vi "DialogCreateClass.vi"(0 "ClassWriterNative.lvclass":refnum<class "ClassWriterNative.lvclass">, 1 "ProjectItem Refnum":refnum<vi>, 5 "error in (no error)":errorcluster) -> (13 "InterfaceToImplement":T3, 14 "Reference out":refnum<class "ClassWriterNative.lvclass">, 15 "Cancelled":bool, 16 "CreateClassData":T4, 17 "DesignPatternsToAddAfterCreation":string[](array[string]), 18 "ChangeProviderRequested":string, 19 "error out":errorcluster)   [LabVIEW 2020, in "ClassWriterNative.lvclass"]
uses:
  <resource>/Framework/Providers/Open_GDS/ClassProviders/Provider_LvNativeClass/ClassWriterNative_class/ClassWriterNative.lvclass
  <resource>/Framework/Providers/Open_GDS/ClassProviders/Provider_BaseClassInterface/CreateClassData.ctl
  <resource>/Framework/Providers/Open_GDS/ClassProviders/Provider_BaseClassInterface/ClassWriter_class/InterfacesToImplement.ctl
  <resource>/Framework/Providers/Open_GDS/ClassProviders/Common/ScriptingFunctions/Scripting_ConnectorPanePatternType.ctl
  <resource>/Framework/Providers/Open_GDS/ClassProviders/Provider_BaseClassInterface/ClassTemplateType.ctl
  <resource>/Framework/Providers/Open_GDS/ClassProviders/Common/InterfaceLibrary/InterfaceInfo.ctl
  <resource>/Framework/Providers/Open_GDS/ClassProviders/Common/LvClass_class/GDSLvClass_ClassMethodInfo.ctl
  <vilib>/Utility/miscctls.llb/LVRectTypeDef.ctl
  <resource>/Framework/Providers/Open_GDS/ClassProviders/Provider_EndevoGOOP400/EndevoG4ProviderName.ctl
  <vilib>/Utility/miscctls.llb/LVPointTypeDef.ctl
  <vilib>/picture/picture.llb/imagedata.ctl
  <vilib>/Utility/miscctls.llb/LVNodeAndColumnTypeDef.ctl
  <vilib>/Utility/miscctls.llb/LVRowAndColumnUnsignedTypeDef.ctl
  dffca1d0-6338-4fa8-b857-2ce53b536d3f.vi
  <resource>/Framework/Providers/Open_GDS/ClassProviders/Provider_BaseClassInterface/ClassWriter_class/ClassWriter.lvclass
  <resource>/Framework/Providers/Open_GDS/ClassProviders/Common/InterfaceLibrary/InterfaceLibrary.lvlib
panel:
  in  "Help":bool
  in  "_HelpCreateClass":bool
  out "IconSelection":picture
  out "Icon":picture
  in  "ConnectorPanePattern":T1 caption="Connector Pane" items=["4x4x4", "5x6x5", "6x8x6"]
  in  "ModifyTemplates":bool
  in  "AddDesignPattern":bool caption="DESIGN PATTERN"
  out "ProductPicture":picture
  out "TriggerSuffixChange":string
  in  "_CurrentClassProvider":u16(ring) caption="Class Provider To Use" items=["EndevoGOOP300", "Endevo LabVIEW Native", "EndevoGOOP400", "OpenG100"]
  in  "_UseLLB":bool
  out "DupPath":bool
  in  "_ClassType":i32(listbox) caption="Class Templates"
  in  "_ClassFolderSuffix":string caption="Class Folder Suffix"
  in  "_ClassName":string caption="Class Name"
  in  "_ClassDescription":string caption="Class Description"
  in  "_ClassFolder":path caption="Save Class To.."
  in  "_SelectParentClass":string(tree)="Derived Class" caption="Select Parent Class"
  in  "CreateInterfaceMethods":T2(ring)
  in  "InterfaceFilter":string caption="Filter"
  in  "_SelectInterfaceClass":i32[](listbox) caption="Select Parent Interface(s) (ctrl+click to do multiple Selection)"
  in  "_Cancel":bool
  in  "_CreateClass":bool
  out "DesignPatternDescription":string caption="Design Pattern Description"
  in  "DesignPatternList":i32(listbox) caption="Design Patterns"
  # "DESIGN PATTERNS SELECTION"
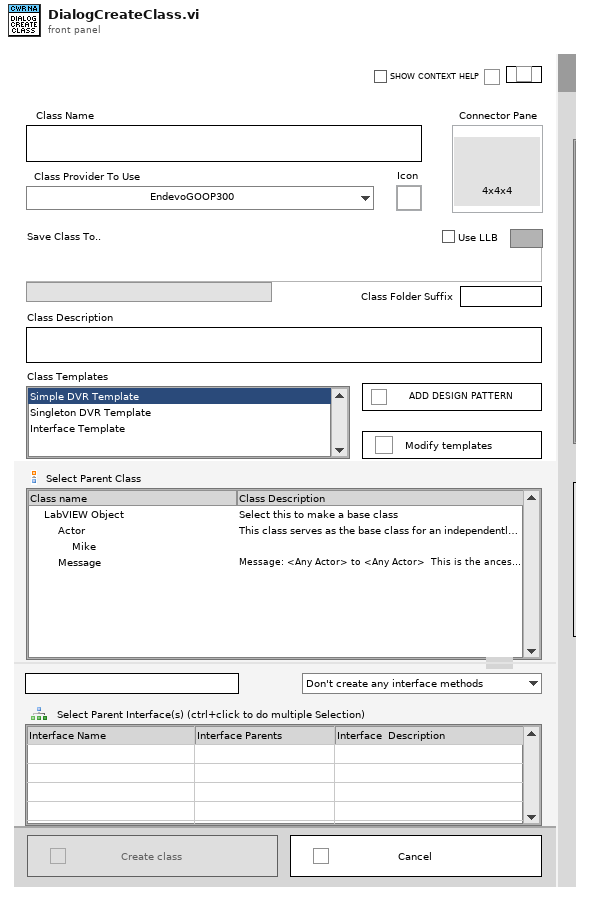
[diagram p1: front panel]
types:
  T1 = typedef "Scripting_ConnectorPanePatternType.ctl" = u16
  T2 = enum16{"Don't create any interface methods", "Create some interface methods", "Create all interface methods"}
  T3 = typedef "ClassWriter.lvclass/InterfacesToImplement.ctl" = cluster{"InterfacePath":path[], "CreateMethods":bool, "MethodsPerInterface(Empty=>All)":cluster{"Methods":string[]}[]}
  T4 = typedef "ClassWriter.lvclass/CreateClassData.ctl" = cluster{"ClassName":string, "ClassFolder":path, "ClassDescription":string, "ClassTemplateOptions":string, "BaseClass(ProjectStringPath or LvClassFilePath)":variant, "ExtraCreateParameters":variant, "FolderSuffix":string}
  T5 = cluster{"Font Name":string, "Size":u16, "Bold":bool, "Italic":bool, "Underline":bool, "Strikeout":bool, "Color":u32}
  T6 = typedef "LVRectTypeDef.ctl" = cluster{"Left":i16, "Top":i16, "Right":i16, "Bottom":i16}
  T7 = typedef "ClassWriter.lvclass/ClassTemplateType.ctl" = cluster{"TemplateIdName":string, "TemplateUserDialogName":string, "OnlySubClassTemplate":bool, "CanDeriveFromTheseTemplateIDs":string[], "ClassSuffix":string, "Description":string, "LvLibTemplate":bool}
  T8 = typedef "InterfaceLibrary.lvlib/InterfaceInfo.ctl" = cluster{"Name(Short if no Conflicts)":string, "FullQualifierName":string, "Description":string, "Path":path, "ParentInterfaceNames(Short if no Conflitcs)":string[], "ParentInterfaceFullQualifierNames":string[], "IconPath":path, "Methods":T9[]}
  T9 = typedef "GDSLvClass_ClassMethodInfo.ctl" = cluster{"Name":string, "Descriptions":string, "RelativePath":path, "SourceScope":enum32{"invalid scope", "public", "private", "protected", "community"}, "MustOverride":bool, "VirtualFolderLocation":string[]}
  T10 = cluster{"Cancel":bool, "OtherTemplates":string[], "BaseClasses":path[], "Templates":T7[], "BaseObjectTag":string, "ClassType(Template)":string, "BaseClassToUse":path, "DeriveFromClass":path, "OpenG":bool, "Derived":bool, "DeriveFromClassRef":refnum<vi>, "ClassPaths":path[], "DesignPatternsVisible":bool, "ClassProviderName":string, "ClassTemplateUsed":string, "PlugInIDs":string[], "DPDescriptions":string[], "DpDependencies":cluster{"DependenciesID":string[]}[], "DPs":string[], "InitDerived":bool, "ClassFolderSuffix":string, "ChangeProviderTo":string, "ClassTags":string[], "LLB_Allowed":bool, "StartFolder":path, "SplitterMouseDown":bool, "InterfaceIcons":path[], "InterfaceInfo":T8[], "OldBnds":T6, "BondsChanged":bool, "ClassTemplateIndex":i32[], "StartBnds":T6}
  T11 = typedef "EndevoG4ProviderName.ctl" = enum16{"EndevoGOOP400"}
  T12 = typedef "LVPointTypeDef.ctl" = cluster{"Horizontal":i16, "Vertical":i16}
  T13 = typedef "imagedata.ctl" = cluster{"image type":i32, "image depth":i32, "image":u8[], "mask":u8[], "colors":u32[], "Rectangle":cluster{"left":i16, "top":i16, "right":i16, "bottom":i16}}
  T14 = typedef "LVNodeAndColumnTypeDef.ctl" = cluster{"Node":string, "Column":i32}
  T15 = typedef "LVRowAndColumnUnsignedTypeDef.ctl" = cluster{"Row":u32, "Column":u32}
  T16 = enum8{"Enabled", "Disabled", "Disabled and Grayed Out"}
  T17 = typedef "GDSLvCLass_ClassSettingsType.ctl" = cluster{"ClassProviderName":string, "ClassTemplateUsed":string, "ClassTemplateVersion":string, "ClassDescription":string, "PlugIns":T18[], "ConnectorPanePattern":string}
  T18 = typedef "GDSLvClass_PlugIn.ctl" = cluster{"Type":T19, "ID":string, "Version":string, "Path":path, "Name":string, "Data":variant}
  T19 = typedef "GDSLvClass_PlugInTypes.ctl" = enum16{"DesignPattern", "MethodTypes"}
  T20 = typedef "BaseProvider_IniFileSettings.ctl" = cluster{"ClassFolderSuffix":string, "InterfaceFolderSuffix":string, "InterfaceIcon":string}
  T21 = enum32{"Invalid", "Standard", "Closed", "Hidden", "Minimized", "Maximized"}
  T22 = typedef "GOOP_WireConfigurationType.ctl" = cluster{"Edge thickness":i32, "Edge color":u32, "Center thickness":i32, "Center pattern":T23, "CenterColor1":u32, "CenterColor2":u32, "Tunnels and terminals colors":u32}
  T23 = typedef "GOOP_WirePattern.ctl" = enum16{"Solid", "Large dash", "Small dash"}
  T24 = typedef "LVPoint32TypeDef.ctl" = cluster{"Horizontal":i32, "Vertical":i32}
  T25 = typedef "DesignPatternsData.ctl" = cluster{"Type":string, "Patterns":cluster{"ID":string, "Path":path, "Name":string, "Desc":string, "Version":string, "DependenciesID":string[], "OnlyOne":bool}[]}
  T26 = cluster{"ID":string, "Path":path, "Name":string, "Desc":string, "Version":string, "DependenciesID":string[], "OnlyOne":bool}[]
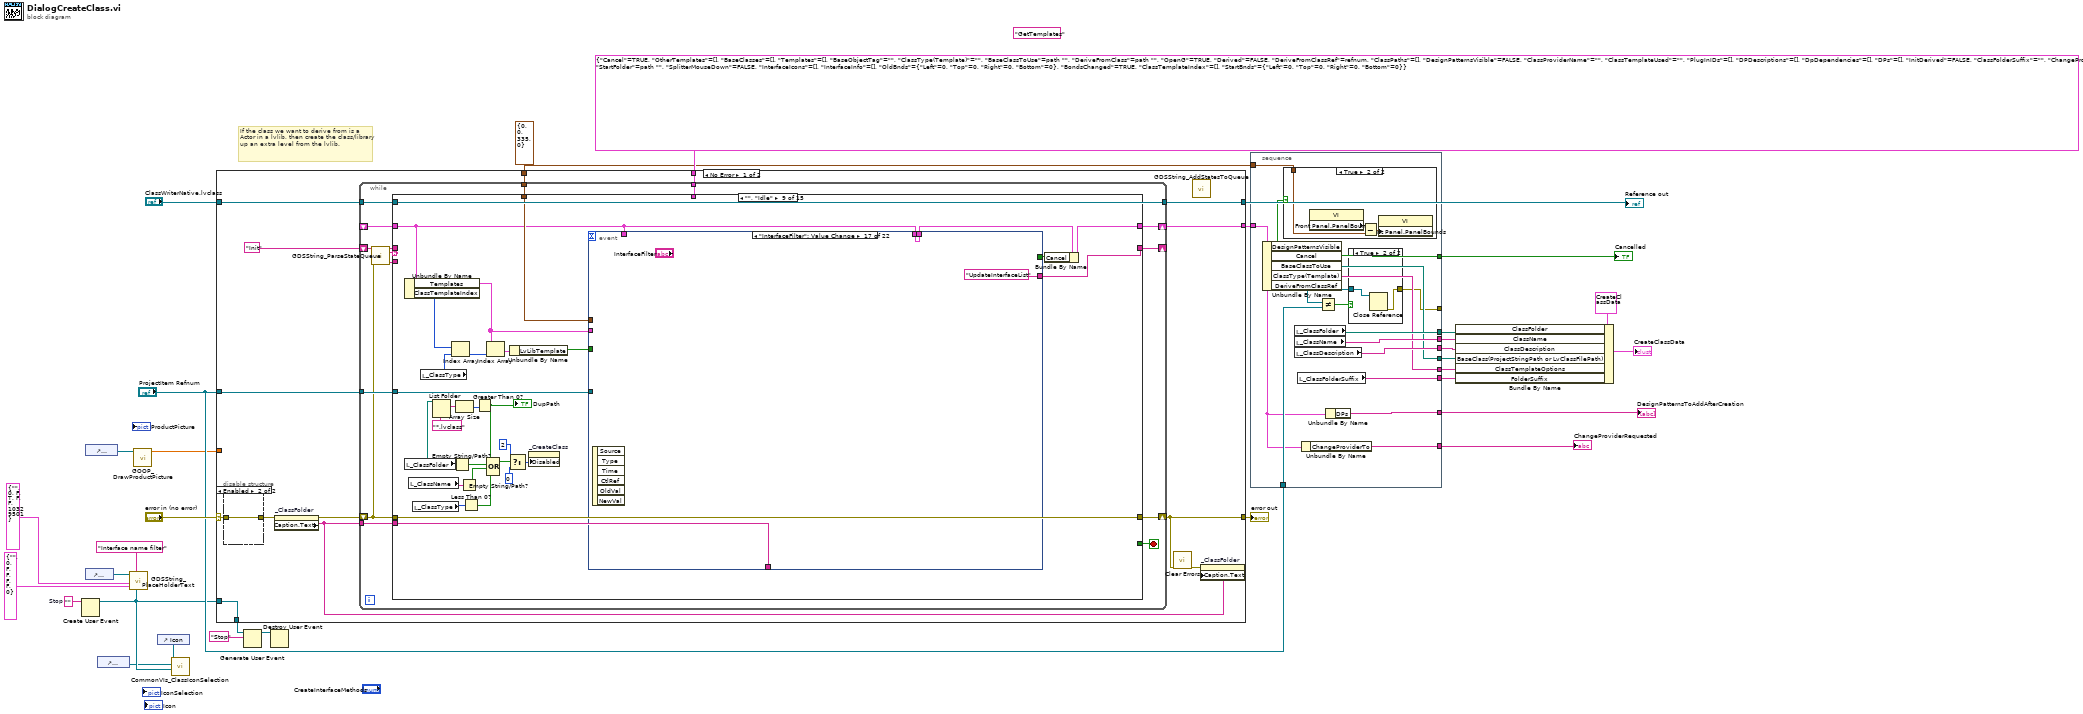
[diagram p0: block diagram]
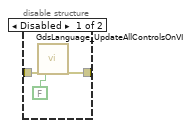
[diagram p4: hidden frame]
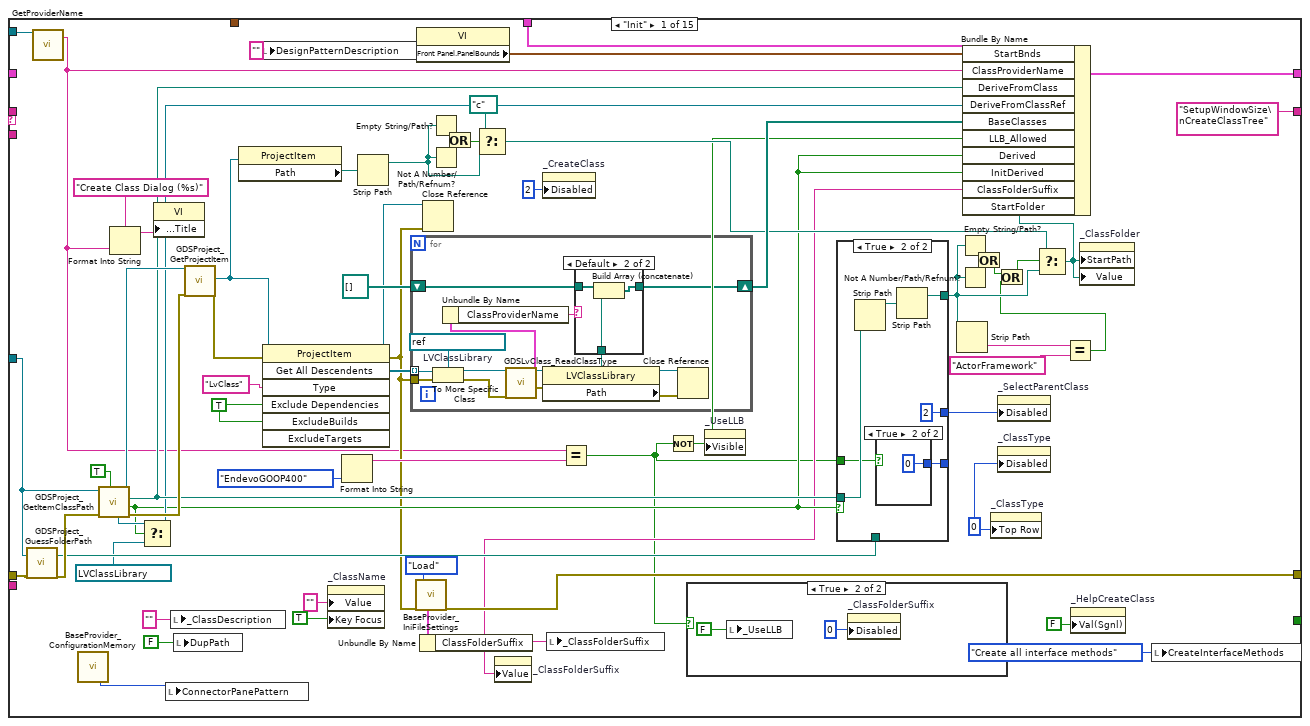
[diagram p5: hidden frame]
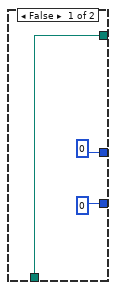
[diagram p8: hidden frame]
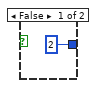
[diagram p9: hidden frame]
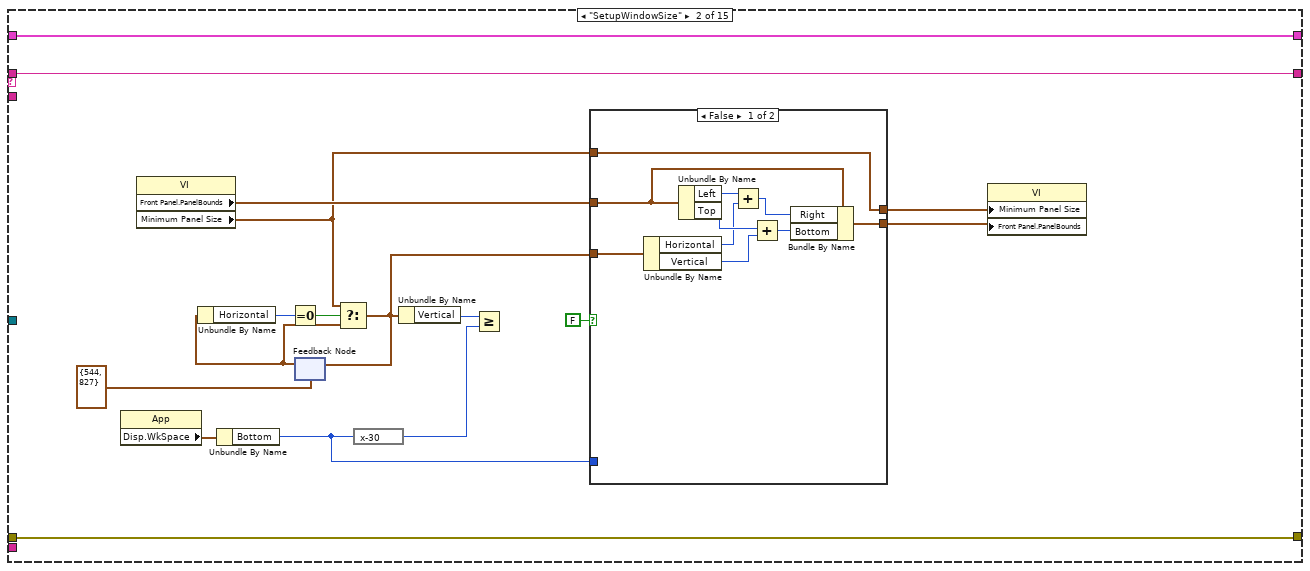
[diagram p10: hidden frame]
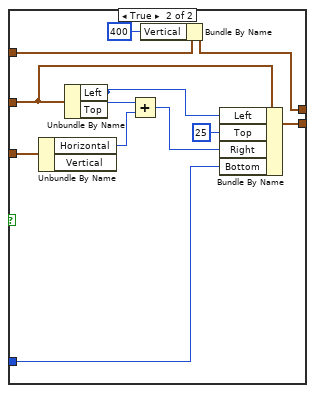
[diagram p11: hidden frame]
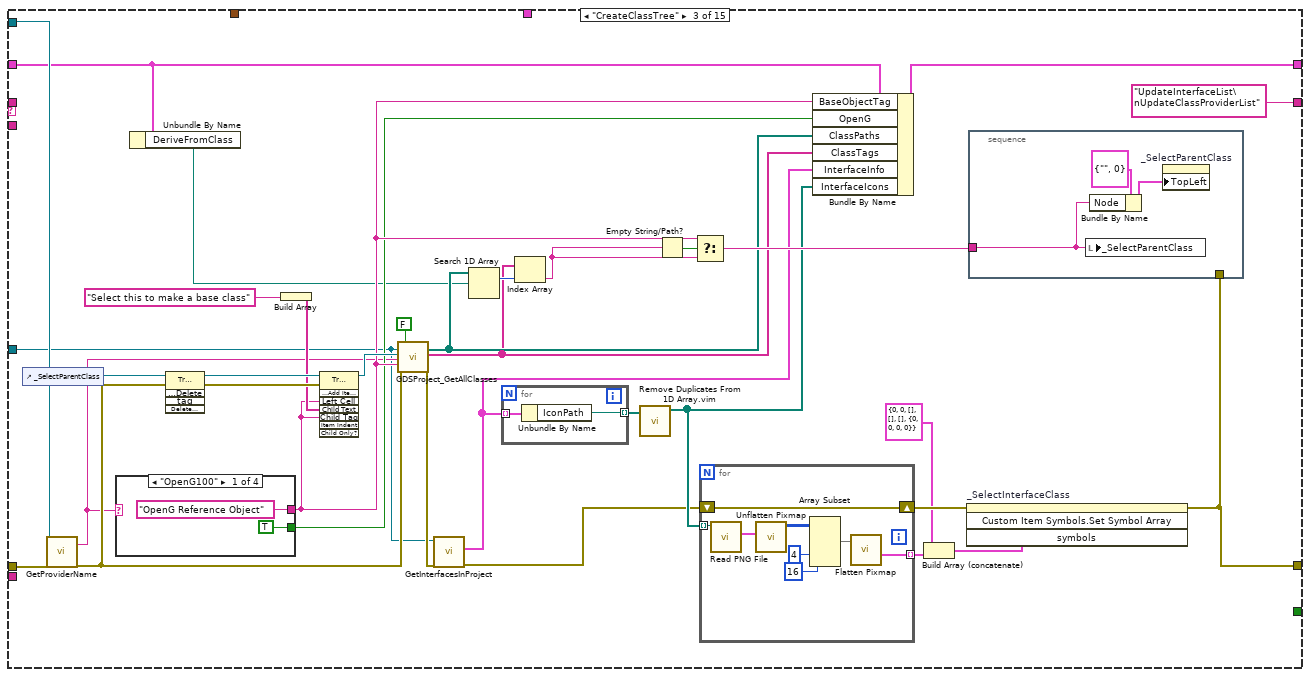
[diagram p12: hidden frame]
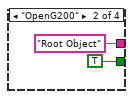
[diagram p13: hidden frame]
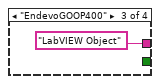
[diagram p14: hidden frame]
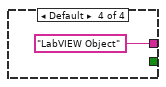
[diagram p15: hidden frame]
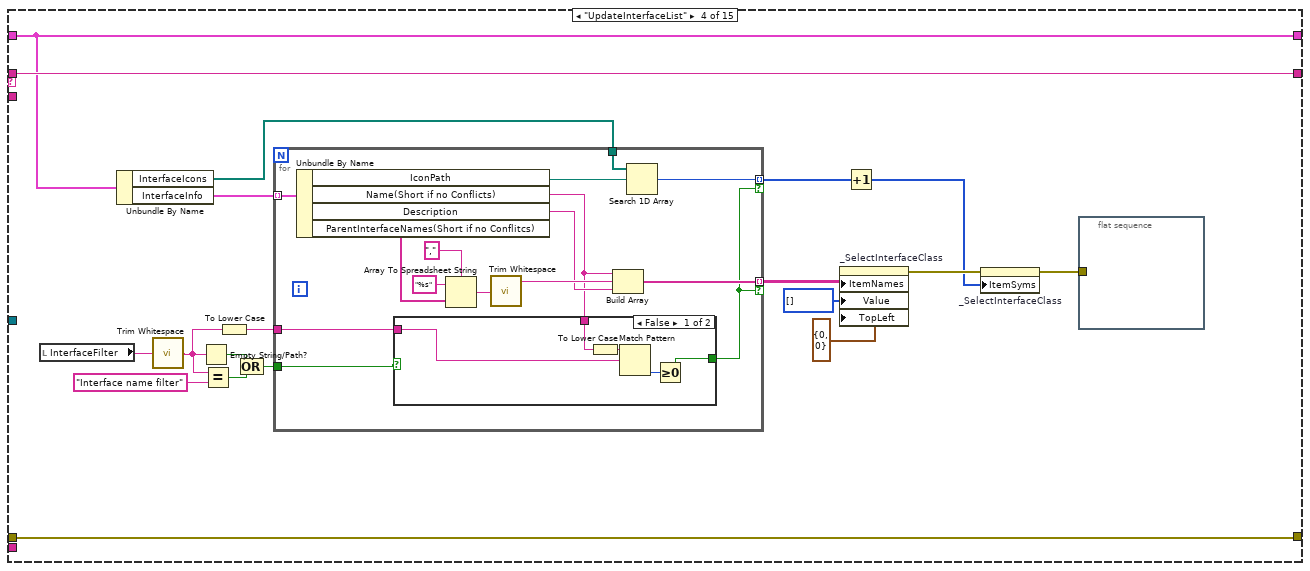
[diagram p16: hidden frame]
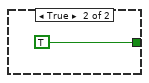
[diagram p17: hidden frame]
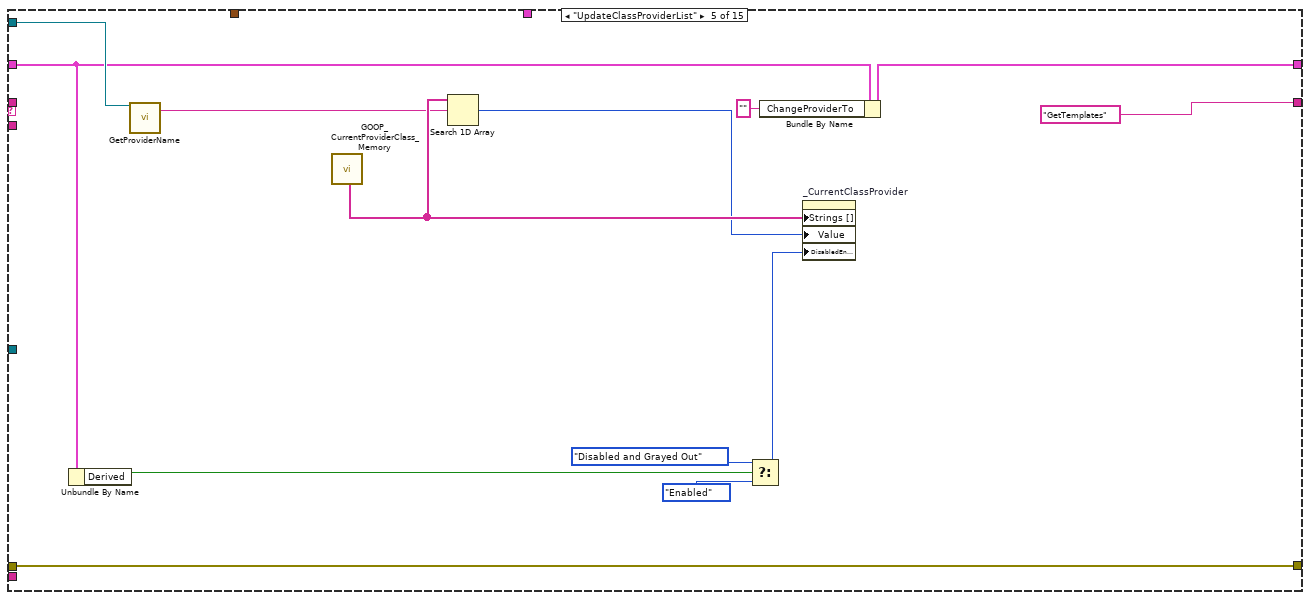
[diagram p18: hidden frame]
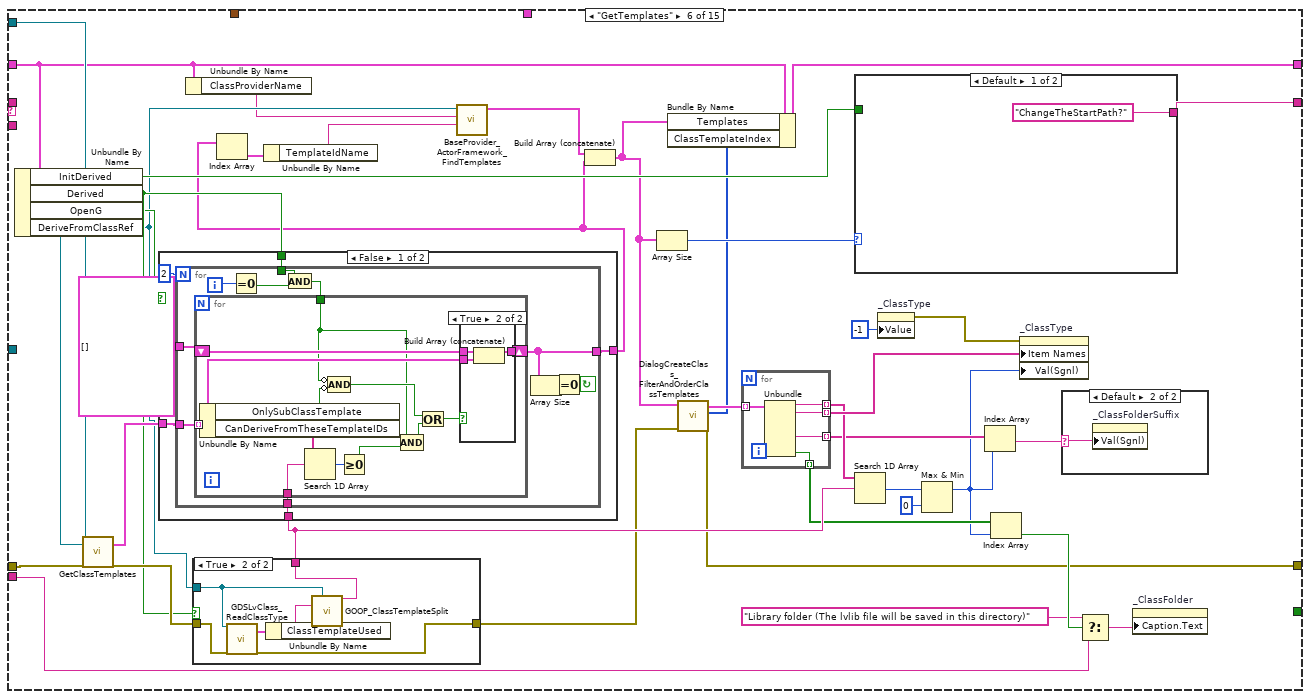
[diagram p19: hidden frame]
diagram:
  w2 = ""  # Stop
  w17 = T6 {"Left"=0, "Top"=0, "Right"=335, "Bottom"=0} ("Rect")
  (unwired) "GetTemplates"
  # "If the class we want to derive from is a\nActor in a lvlib, then create the class/library\nup an extra level from the lvlib."
  n1 = Create User Event(user event datatype=w2) -> (user event=w5:refnum<user-event>)  [unwired: 1 in, 1 out]
  n2 = control-ref of="InterfaceFilter"() -> (w11:refnum<vi>)
  n3 = control-ref of="ProductPicture"() -> (w13:refnum<vi>)
  n4 = control-ref of="IconSelection"() -> (w3:refnum<vi>)
  n5 = call <resource>:"GDSString_PlaceHolderText.vi"("BooleanUserEventToStopPlaceHolderVI"=w5, "PlaceholderText"="Interface name filter" ("InterfaceFilter"), "PlaceholderTextFont(Grey,Italic)"=T5 {"Font Name"="", "Size"=0, "Bold"=FALSE, "Italic"=TRUE, "Underline"=FALSE, "Strikeout"=FALSE, "Color"=10329501}, "NormalTextFont(Black)"=T5 {"Font Name"="", "Size"=0, "Bold"=FALSE, "Italic"=FALSE, "Underline"=FALSE, "Strikeout"=FALSE, "Color"=0}, "PlaceholderStringRef"=w11) -> ()  [unwired: 6 in, 1 out]
  n6 = call <resource>:"GOOP_DrawProductPicture.vi"("ProductPictureControl"=w13) -> ("Zoom Factor"=w12:sgl)  [unwired: 10 in]
  n7 = control-ref of="Icon"() -> (w4:refnum<vi>)
  n8 = call <resource>:"CommonVIs_ClassIconSelection.vi"("Icon"=w4, "Messages(Stop or Empty string will stop this VI)"=w5, "IconSelection"=w3) -> ()  [unwired: 9 in]
  n9 = case shown="No Error" "error in (no error)" {
    selector: "error in (no error)" -> [w41 w1013]
    tunnel: "ClassWriterNative.lvclass" -> [w45 w1012]
    tunnel: [w34 w1013] -> w31
    tunnel: [w46 w1012] -> w29
    tunnel: T10 {"Cancel"=TRUE, "OtherTemplates"=[], "BaseClasses"=[], "Templates"=[], "BaseObjectTag"="", "ClassType(Template)"="", "BaseClassToUse"=path "", "DeriveFromClass"=path "", "OpenG"=TRUE, "Derived"=FALSE, "DeriveFromClassRef"=refnum, "ClassPaths"=[], "DesignPatternsVisible"=FALSE, "ClassProviderName"="", "ClassTemplateUsed"="", "PlugInIDs"=[], "DPDescriptions"=[], "DpDependencies"=[], "DPs"=[], "InitDerived"=FALSE, "ClassFolderSuffix"="", "ChangeProviderTo"="", "ClassTags"=[], "LLB_Allowed"=FALSE, "StartFolder"=path "", "SplitterMouseDown"=FALSE, "InterfaceIcons"=[], "InterfaceInfo"=[], "OldBnds"={"Left"=0, "Top"=0, "Right"=0, "Bottom"=0}, "BondsChanged"=TRUE, "ClassTemplateIndex"=[], "StartBnds"={"Left"=0, "Top"=0, "Right"=0, "Bottom"=0}} ("output cluster") -> [w44 _]
    tunnel: "ProjectItem Refnum" -> [w43 _]
    tunnel: [w42 _] -> w27
    tunnel: w17 -> [w40 _]
    tunnel: w12 -> [_ _]
    tunnel: w5 -> [w36 w1011]
    tunnel: [w36 w1011] -> w8
    frame No Error {
      n10 = disable-structure shown="Enabled" {
        disable-tunnel: w41 -> [w49 w50]
        disable-tunnel: [w47 w50] -> w39
        frame Disabled {
          n11 = call <resource>:"GdsLanguage_UpdateAllControlsOnVI.vi"("error in (no error)"=w49, "CreateLanguageFile(Use this to create a languageFile)"=FALSE) -> ("error out"=w47:errorcluster)  [unwired: 16 in, 1 out]
        }
        frame Enabled {
        }
      }
      n12 = property on="_ClassFolder" class="Path"(error in=w39) -> (error out=w38:errorcluster, "Caption.Text"=w37:string)  [unwired: 1 in, 1 out]
      n13 = while {
        shift-right: [w64] -> w34
        shift-left: w38 -> [w56]
        shift-right: [w54] -> _
        shift-left: "Init" -> [w57]
        shift-right: [w60] -> w42
        shift-left: _ -> [w65]
        tunnel: w45 -> [w63]
        tunnel: [w63] -> w46
        tunnel: w44 -> [w62]
        tunnel: w43 -> [w61]
        tunnel: w40 -> [w59]
        tunnel: w37 -> [w58]
        stop <- w55 stop-if-true
        n14 = call <resource>:"GDSString_ParseStateQueue.vi"("State Queue"=w57, "Error In (no error)"=w56) -> ("Remaining States"=w52:string, "Current State"=w53:string, "Arguments"=w51:string)  [unwired: 9 in, 2 out]
        n15 = case shown="\"\", \"Idle\"" w53 {
          tunnel: w65 -> [_ w176 w221 w267 w293 w320 w401 w427 w434 w809 w838 w899 w984 w1006 w1010]
          tunnel: [w127 w176 w223 w267 w292 w339 w401 w427 w454 w824 w837 w926 w984 w1006 w1010] -> w60
          tunnel: w56 -> [w104 w175 w226 w268 w302 w334 w397 w426 w457 w826 w847 w917 w990 _ w1009]
          tunnel: [w83 w175 w200 w268 w302 w305 w397 w426 w457 w826 w846 w916 w990 errorcluster {"status"=TRUE, "code"=1, "source"="Invalid Case"} ("error out") w1009] -> w64
          tunnel: w63 -> [w96 _ w229 _ w295 w338 _ _ _ _ _ _ _ _ _]
          tunnel: ["SetupWindowSize\nCreateClassTree" w174 "UpdateInterfaceList\nUpdateClassProviderList" w269 "GetTemplates" w340 "Idle" "Idle" w455 w825 "Idle" "GetInterfaceSettings" "Exit" "Exit" "Exit"] -> w54
          tunnel: w62 -> [w126 _ _ _ _ _ _ _ _ _ _ _ _ _ _]
          tunnel: w61 -> [w102 _ w207 _ _ _ _ _ w439 _ _ _ _ _ _]
          tunnel: w59 -> [_ _ _ _ _ _ _ _ w437 _ _ _ _ _ _]
          tunnel: w58 -> [_ _ _ _ _ w313 _ _ w436 w811 _ _ _ _ _]
          tunnel: [_ _ _ _ _ _ _ _ _ _ _ _ _ TRUE TRUE] -> w55
          tunnel: w52 -> [_ w174 _ w269 _ _ _ _ _ w825 _ _ _ _ _]
          tunnel: w51 -> [_ _ _ _ _ _ _ _ _ _ _ _ _ _ _]
          frame "Init" {
            w91 = 0 ("Top Row")
            w95 = TRUE ("ExcludeDependencies")
            n16 = call <resource>:"GDSProject_GuessFolderPath.vi"("ProjectItem"=w102, "error in (no error)"=w104) -> ("Path"=w101:path, "error out"=w103:errorcluster)  [unwired: 14 in, 2 out]
            n17 = call-dynamic "GetProviderName.vi"("ClassWriterNative in"=w96) -> ("ProviderName"=w80:string)  [unwired: 16 in, 2 out]
            n18 = call <resource>:"BaseProvider_ConfigurationMemory.vi"() -> ("PatternOut"=w67:T1)  [unwired: 13 in, 6 out]
            n19 = call <resource>:"GDSProject_GetItemClassPath.vi"("ReturnRefToClass(False)"=TRUE, "error in"=w103, "ProjectItemRefIn"=w102) -> ("error out"=w123:errorcluster, "LvCLassFound"=w86:bool, "Path"=w99:path, "ProjectItemRefOut"=w121:refnum<vi>, "LvClassRef"=w90:refnum<vi>)  [unwired: 3 in, 1 out]
            n20 = Format Into String(format string="Create Class Dialog (%s)", w80) -> (resulting string=w98:string)  [unwired: 2 in, 1 out]
            n21 = Select(t=w90, s=w86, f=refnum<vi> refnum) -> (s? t:f=w89:refnum<vi>)
            n22 = property class="VI"("Front Panel.Title"=w98) -> ()  [unwired: 2 in, 2 out]
            n23 = local write "ConnectorPanePattern"(w67) -> ()
            n24 = local write "_ClassDescription"("" ("Class description")) -> ()
            n25 = local write "DupPath"(FALSE ("DupPath")) -> ()
            n26 = call <resource>:"GDSProject_GetProjectItem.vi"("ProjectItemToSearchFrom"=w121, "error in (no error)"=w123) -> ("ProjectItemFound"=w111:refnum<vi>, "error out"=w122:errorcluster)  [unwired: 14 in, 2 out]
            n27 = property class="ProjectItem"(reference=w111) -> ("Path"=w106:path)  [unwired: 1 in, 2 out]
            n28 = local write "DesignPatternDescription"("" ("DesignPatternDescription")) -> ()
            n29 = invoke class="ProjectItem" method="Get All Descendents"(reference=w111, error in=w122, "Type"="LvClass" ("x"), "Exclude Dependencies"=w95, "ExcludeBuilds"=w95) -> (reference out=w118:refnum<vi>, error out=w83:errorcluster, "All Descendents"=w120:refnum<vi>[])  [unwired: 2 in, 4 out]
            n30 = property on="_ClassName" class="Str"("Value"="" ("Class name"), "Key Focus"=TRUE) -> ()  [unwired: 2 in, 2 out]
            n31 = Format Into String(EndevoG4ProviderName."EndevoGOOP400" ("ProviderName")) -> (resulting string=w84:string)  [unwired: 3 in, 1 out]
            n32 = Strip Path(path=w106) -> (stripped path=w105:path)  [unwired: 1 out]
            n33 = for {
              tunnel: w120 -> [w144] mode=indexing
              shift-right: [w140] -> w117
              shift-left: path[] [] -> [w139]
              tunnel: w83 -> [w135]
              w143 = refnum<vi> refnum  # LVClassLibrary
              n34 = To More Specific Class(target class=w143, reference=w144, error in=w135) -> (specific class reference=w142:refnum<vi>, error out=w141:errorcluster)
              n35 = call <resource>:"GDSLvClass_ReadClassType.vi"("Class Refnum In"=w142, "error in (no error)"=w141) -> ("Class Refnum Out"=w137:refnum<vi>, "ClassSettings"=w134:T17, "error out"=w138:errorcluster)  [unwired: 15 in]
              n36 = Unbundle By Name(w134) -> ("ClassProviderName"=w133:string)
              n37 = property class="LVClassLibrary"(reference=w137, error in=w138) -> (reference out=w131:refnum<vi>, error out=w132:errorcluster, "Path"=w136:path)
              n38 = case shown="Default" w133 {
                tunnel: [w145 w148] -> w140
                tunnel: w139 -> [w145 w147]
                tunnel: w136 -> [_ w146]
                frame "" {
                }
                frame Default {
                  n39 = Build Array (concatenate)(w147, w146) -> (w148:path[])
                }
              }
              n40 = Close Reference(reference=w131, error in (no error)=w132) -> ()  [unwired: 1 out]
            }
            n41 = call <resource>:"BaseProvider_IniFileSettings.vi"("error in (no error)"=w83, "Action"=enum16{"Read", "Load", "Save"}."Load") -> ("IniFileSettings"=w81:T20)  [unwired: 16 in, 1 out]
            n42 = property class="VI"() -> ("Front Panel.PanelBounds"=w66:T6)  [unwired: 2 in, 2 out]
            n43 = Unbundle By Name(w81) -> ("ClassFolderSuffix"=w79:string)
            n44 = Close Reference(reference=w118, error in (no error)=w83) -> ()  [unwired: 1 out]
            n45 = Empty String/Path?(string/path=w105) -> (empty?=w107:bool)
            n46 = Not A Number/Path/Refnum?(number/path/refnum=w105) -> (NaN/Path/Refnum?=w108:bool)
            n47 = Or(x=w107, y=w108) -> (x .or. y?=w109:bool)
            n48 = Select(t=path "c:/", s=w109, f=w105) -> (s? t:f=w93:path)
            n49 = property on="_ClassFolderSuffix" class="Str"("Value"=w79) -> ()  [unwired: 2 in, 2 out]
            n50 = property on="_CreateClass" class="Bool"("Disabled"=u8 2) -> ()  [unwired: 2 in, 2 out]
            n51 = local write "_ClassFolderSuffix"(w79) -> ()
            n52 = Equal?(x=w80, y=w84) -> (x = y?=w77:bool)
            n53 = Not(x=w77) -> (.not. x?=w78:bool)
            n54 = case shown="True" w77 {
              frame False {
              }
              frame True {
                n55 = local write "_UseLLB"(FALSE ("_UseLLB")) -> ()
                n56 = property on="_ClassFolderSuffix" class="Str"("Disabled"=u8 0) -> ()  [unwired: 2 in, 2 out]
              }
            }
            n57 = property on="_UseLLB" class="Bool (strict)"("Visible"=w78) -> ()  [unwired: 2 in, 2 out]
            n58 = case shown="True" w86 {
              tunnel: w99 -> [_ w156]
              tunnel: [w150 w154] -> w75
              tunnel: [u8 0 ("Disabled") w157] -> _
              tunnel: w101 -> [w150 _]
              tunnel: w77 -> [_ w153]
              tunnel: [u8 0 ("Disabled") u8 2 ("Disabled")] -> w92
              frame False {
              }
              frame True {
                n59 = Strip Path(path=w156) -> (stripped path=w155:path)  [unwired: 1 out]
                n60 = case shown="True" w153 {
                  tunnel: [u8 2 ("Disabled") u8 0 ("Disabled")] -> w157
                  frame False {
                  }
                  frame True {
                  }
                }
                n61 = Strip Path(path=w155) -> (stripped path=w154:path)  [unwired: 1 out]
              }
            }
            n62 = Strip Path(path=w75) -> (name=w74:string)  [unwired: 1 out]
            n63 = Empty String/Path?(string/path=w75) -> (empty?=w113:bool)
            n64 = Not A Number/Path/Refnum?(number/path/refnum=w75) -> (NaN/Path/Refnum?=w112:bool)
            n65 = Or(x=w113, y=w112) -> (x .or. y?=w72:bool)
            n66 = property on="_ClassType" class="LstBox (strict)"("Top Row"=w91) -> ()  [unwired: 2 in, 2 out]
            n67 = property on="_SelectParentClass" class="Tree (strict)"("Disabled"=w92) -> ()  [unwired: 2 in, 2 out]
            n68 = property on="_ClassType" class="LstBox (strict)"("Disabled"=w91) -> ()  [unwired: 2 in, 2 out]
            n69 = Equal?(x=w74, y="ActorFramework") -> (x = y?=w71:bool)
            n70 = Or(x=w72, y=w71) -> (x .or. y?=w70:bool)
            n71 = Select(t=w93, s=w70, f=w75) -> (s? t:f=w76:path)
            n72 = Bundle By Name(cluster=w126, "StartBnds"=w66, "ClassProviderName"=w80, "DeriveFromClass"=w99, "DeriveFromClassRef"=w89, "BaseClasses"=w117, "LLB_Allowed"=w78, "Derived"=w86, "InitDerived"=w86, "ClassFolderSuffix"=w79, "StartFolder"=w76) -> (w127:T10)
            n73 = property on="_HelpCreateClass" class="Bool (strict)"("Val(Sgnl)"=FALSE ("Value (Signaling)")) -> ()  [unwired: 2 in, 2 out]
            n74 = property on="_ClassFolder" class="Path"("StartPath"=w76, "Value"=w76) -> ()  [unwired: 2 in, 2 out]
            n75 = local write "CreateInterfaceMethods"(T2."Create all interface methods" ("CreateInterfaceMethods")) -> ()
          }
          frame "SetupWindowSize" {
            n76 = property class="App"() -> ("Disp.WkSpace"=w173:T6)  [unwired: 2 in, 2 out]
            n77 = property class="VI"() -> ("Front Panel.PanelBounds"=w172:T6, "Minimum Panel Size"=w161:T12)  [unwired: 2 in, 2 out]
            n78 = Unbundle By Name(w173) -> ("Bottom"=w164:i16)
            n79 = feedback #1(T12 {"Horizontal"=544, "Vertical"=827} ("Minimum Panel Size")) -> (w169:T12)
            n80 = Unbundle By Name(w169) -> ("Horizontal"=w171:i16)
            n81 = Equal To 0?(x=w171) -> (x = 0?=w170:bool)
            n82 = Select(t=w161, s=w170, f=w169) -> (s? t:f=w168:T12)
            n83 = feedback-in #1(w168) -> ()
            n84 = expression code="x-30"(w164) -> (w166:i16)
            n85 = Unbundle By Name(w168) -> ("Vertical"=w167:i16)
            n86 = Greater Or Equal?(x=w167, y=w166) -> ()  [unwired: 1 out]
            n87 = case shown="False" FALSE {
              tunnel: w172 -> [w179 w194]
              tunnel: w168 -> [w182 w197]
              tunnel: [w178 w195] -> w165
              tunnel: w164 -> [_ w190]
              tunnel: [w177 w188] -> w162
              tunnel: w161 -> [w177 w189]
              frame False {
                n88 = Unbundle By Name(w182) -> ("Horizontal"=w184:i16, "Vertical"=w186:i16)
                n89 = Unbundle By Name(w179) -> ("Left"=w183:i16, "Top"=w185:i16)
                n90 = Add(x=w183, y=w184) -> (x+y=w181:i16)
                n91 = Add(x=w185, y=w186) -> (x+y=w180:i16)
                n92 = Bundle By Name(cluster=w179, "Right"=w181, "Bottom"=w180) -> (w178:T6)
              }
              frame True {
                n93 = Unbundle By Name(w197) -> ("Horizontal"=w196:i16)  [unwired: 1 out]
                n94 = Unbundle By Name(w194) -> ("Left"=w193:i16)  [unwired: 1 out]
                n95 = Add(x=w193, y=w196) -> (x+y=w192:i16)
                n96 = Bundle By Name(cluster=w189, "Vertical"=i16 400) -> (w188:T12)
                n97 = Bundle By Name(cluster=w194, "Left"=w193, "Top"=i16 25, "Right"=w192, "Bottom"=w190) -> (w195:T6)
              }
            }
            n98 = property class="VI"("Minimum Panel Size"=w162, "Front Panel.PanelBounds"=w165) -> ()  [unwired: 2 in, 2 out]
          }
          frame "CreateClassTree" {
            n99 = control-ref of="_SelectParentClass"() -> (w230:refnum<vi>)
            n100 = call-dynamic "GetProviderName.vi"("ClassWriterNative in"=w229, "error in (no error)"=w226) -> ("ProviderName"=w209:string, "error out"=w216:errorcluster)  [unwired: 15 in, 1 out]
            n101 = case shown="\"OpenG100\"" w209 {
              tunnel: ["OpenG Reference Object" ("Child Tag") "Root Object" ("Child Tag") "LabVIEW Object" ("Child Tag") "LabVIEW Object" ("Child Tag")] -> w219
              tunnel: [TRUE TRUE _ _] -> w217
              frame "OpenG100" {
              }
              frame "OpenG200" {
              }
              frame "EndevoGOOP400" {
              }
              frame Default {
              }
            }
            n102 = Unbundle By Name(w221) -> ("DeriveFromClass"=w214:path)
            n103 = invoke class="Tree (strict)" method="Edit Tree Items.Delete"(reference=w230, error in=w216) -> (reference out=w228:refnum<vi>, error out=w227:errorcluster)  [unwired: 3 in, 3 out]
            n104 = Build Array("Select this to make a base class" ("Child Tag")) -> (w224:string[])
            n105 = invoke class="Tree (strict)" method="Edit Tree Items.Add Item to End"(reference=w228, error in=w227, "Left Cell"=w219, "Child Text"=w224, "Child Tag"=w219) -> (reference out=w222:refnum<vi>)  [unwired: 3 in, 7 out]
            n106 = call <resource>:"GDSProject_GetAllClasses.vi"("AnyProjectItemRefnum"=w207, "TreeControlRef"=w222, "ClassProviderName"=w209, "RootParentTag"=w219, "error In"=w216, "Interfaces(False)"=FALSE) -> ("ClassPaths"=w215:path[], "ClassTags"=w212:string[], "error out"=w208:errorcluster)  [unwired: 11 in]
            n107 = call <resource>:"GetInterfacesInProject.vi"("error in"=w208, "Project/ProjectItem"=w207) -> ("error out"=w203:errorcluster, "InterfaceInfo"=w206:T8[])  [unwired: 8 in]
            n108 = Search 1D Array(1D array=w215, element=w214) -> (index of element=w213:i32)  [unwired: 1 in]
            n109 = for {
              tunnel: w206 -> [w241] mode=indexing
              tunnel: [w240] -> w205 mode=indexing
              n110 = Unbundle By Name(w241) -> ("IconPath"=w240:path)
            }
            n111 = Index Array(array=w212, index=w213) -> (element=w211:string)
            n112 = call "Remove Duplicates From 1D Array.vim"("array"=w205) -> ("array with duplicates removed"=w204:path[])  [unwired: 10 in]
            n113 = Empty String/Path?(string/path=w211) -> (empty?=w220:bool)
            n114 = Select(t=w219, s=w220, f=w211) -> (s? t:f=w218:string)
            n115 = for {
              tunnel: w204 -> [w239] mode=indexing
              shift-right: [w233] -> w202
              shift-left: w203 -> [w233]
              tunnel: [w232] -> w201 mode=indexing
              n116 = call <vilib>:"Read PNG File.vi"("path to PNG file"=w239) -> ("image data"=w238:T13)  [unwired: 8 in, 2 out]
              n117 = call <vilib>:"Unflatten Pixmap.vi"("image data"=w238) -> ("24-bit pixmap"=w237:u32[][])  [unwired: 4 in, 6 out]
              n118 = Array Subset(array=w237, index (col)=4 ("index"), length (col)=16 ("length")) -> (w234:u32[][])  [unwired: 2 in]
              n119 = call <vilib>:"Flatten Pixmap.vi"("24-bit pixmap"=w234) -> ("image data"=w232:T13)  [unwired: 10 in]
            }
            n120 = Bundle By Name(cluster=w221, "BaseObjectTag"=w219, "OpenG"=w217, "ClassPaths"=w215, "ClassTags"=w212, "InterfaceInfo"=w206, "InterfaceIcons"=w204) -> (w223:T10)
            n121 = Build Array (concatenate)(T13 {"image type"=0, "image depth"=0, "image"=[], "mask"=[], "colors"=[], "Rectangle"={"left"=0, "top"=0, "right"=0, "bottom"=0}} ("image data"), w201) -> (w198:T13[])
            n122 = invoke on="_SelectInterfaceClass" class="MCListbox (strict)" method="Custom Item Symbols.Set Symbol Array"(error in=w202, "symbols"=w198) -> (error out=w200:errorcluster)  [unwired: 2 in, 3 out]
            n123 = stacked-sequence {
              tunnel: w218 -> [w248]
              tunnel: w200 -> [_]
              frame #0 {
                n124 = local write "_SelectParentClass"(w248) -> ()
                n125 = Bundle By Name(cluster=T14 {"Node"="", "Column"=0} ("Top Left Visible Cell"), "Node"=w248) -> (w249:T14)
                n126 = property on="_SelectParentClass" class="Tree (strict)"("TopLeft"=w249) -> ()  [unwired: 2 in, 2 out]
              }
            }
          }
          frame "UpdateInterfaceList" {
            n127 = local read "InterfaceFilter"() -> (w262:string)
            n128 = Unbundle By Name(w267) -> ("InterfaceIcons"=w265:path[], "InterfaceInfo"=w266:T8[])
            n129 = call <vilib>:"Trim Whitespace.vi"("string"=w262) -> ("trimmed string"=w257:string)  [unwired: 1 in]
            n130 = Empty String/Path?(string/path=w257) -> (empty?=w260:bool)
            n131 = Equal?(x=w257, y="Interface name filter" ("InterfaceFilter")) -> (x = y?=w259:bool)
            n132 = To Lower Case(string=w257) -> (all lower case string=w253:string)
            n133 = Compound Arithmetic op=OR(w260, w259) -> (w258:bool)
            n134 = for {
              tunnel: [w280] -> w264 mode=indexing if=w272
              tunnel: w266 -> [w279] mode=indexing
              tunnel: w265 -> [w275]
              tunnel: [w274] -> w252 mode=indexing if=w272
              tunnel: w258 -> [w273]
              tunnel: w253 -> [w270]
              n135 = Unbundle By Name(w279) -> ("IconPath"=w276:path, "Name(Short if no Conflicts)"=w271:string, "Description"=w277:string, "ParentInterfaceNames(Short if no Conflitcs)"=w278:string[])
              n136 = case shown="False" w273 {
                tunnel: [w286 TRUE] -> w272
                tunnel: w271 -> [w289 _]
                tunnel: w270 -> [w288 _]
                frame False {
                  n137 = To Lower Case(string=w289) -> (all lower case string=w285:string)
                  n138 = Match Pattern(string=w285, regular expression=w288) -> (offset past match=w287:i32)  [unwired: 1 in, 3 out]
                  n139 = Greater Or Equal To 0?(x=w287) -> (x >= 0?=w286:bool)
                }
                frame True {
                }
              }
              n140 = Array To Spreadsheet String(delimiter (Tab)=",", array=w278, 3:"%s" ("format string")) -> (spreadsheet string=w282:string)
              n141 = call <vilib>:"Trim Whitespace.vi"("string"=w282) -> ("trimmed string"=w281:string)  [unwired: 1 in]
              n142 = Build Array(w271, w281, w277) -> (w280:string[])
              n143 = Search 1D Array(1D array=w275, element=w276) -> (index of element=w274:i32)  [unwired: 1 in]
            }
            n144 = property on="_SelectInterfaceClass" class="MCListbox (strict)"("ItemNames"=w264, "Value"=i32[] [] ("_SelectInterfaceClass"), "TopLeft"=T15 {"Row"=0, "Column"=0} ("Top Left Visible Cell")) -> (error out=w263:errorcluster)  [unwired: 2 in, 1 out]
            n145 = Increment(x=w252) -> (x+1=w251:i32[])
            n146 = property on="_SelectInterfaceClass" class="MCListbox (strict)"(error in=w263, "ItemSyms"=w251) -> (error out=w254:errorcluster)  [unwired: 1 in, 1 out]
            n147 = flat-sequence {
              tunnel: w254 -> [_]
              frame #0 {
              }
            }
          }
          frame "UpdateClassProviderList" {
            n148 = Unbundle By Name(w293) -> ("Derived"=w299:bool)
            n149 = call-dynamic "GetProviderName.vi"("ClassWriterNative in"=w295) -> ("ProviderName"=w294:string)  [unwired: 16 in, 2 out]
            n150 = call <resource>:"GOOP_CurrentProviderClass_Memory.vi"() -> ("AllClassProviders"=w301:string[])  [unwired: 15 in, 4 out]
            n151 = Search 1D Array(1D array=w301, element=w294) -> (index of element=w300:i32)  [unwired: 1 in]
            n152 = Select(t=T16."Disabled and Grayed Out" ("Disabled"), s=w299, f=T16."Enabled" ("Disabled")) -> (s? t:f=w298:T16)
            n153 = Bundle By Name(cluster=w293, "ChangeProviderTo"="") -> (w292:T10)
            n154 = property on="_CurrentClassProvider" class="Ring (strict)"("Strings []"=w301, "Value"=w300, "DisabledEnum"=w298) -> ()  [unwired: 2 in, 2 out]
          }
          frame "GetTemplates" {
            n155 = Unbundle By Name(w320) -> ("InitDerived"=w326:bool, "Derived"=w333:bool, "OpenG"=w327:bool, "DeriveFromClassRef"=w323:refnum<vi>)
            n156 = call-dynamic "GetClassTemplates.vi"("ClassWriterNative in"=w338, "DerivedFromThisClass(if any)"=w323, "error in (no error)"=w334) -> ("Templates"=w337:T7[], "error out"=w336:errorcluster)  [unwired: 14 in, 1 out]
            n157 = Unbundle By Name(w320) -> ("ClassProviderName"=w319:string)
            n158 = case shown="True" w333 {
              tunnel: w336 -> [w380 w385]
              tunnel: w323 -> [_ w381]
              tunnel: [w380 w384] -> w306
              tunnel: [_ w382] -> w330
              frame False {
              }
              frame True {
                n159 = call <resource>:"GDSLvClass_ReadClassType.vi"("Class Refnum In"=w381, "error in (no error)"=w385) -> ("ClassSettings"=w386:T17, "error out"=w384:errorcluster)  [unwired: 15 in, 1 out]
                n160 = Unbundle By Name(w386) -> ("ClassTemplateUsed"=w383:string)
                n161 = call <resource>:"GOOP_ClassTemplateSplit.vi"("ClassItemRefIn"=w381, "FullClassTemplate"=w383) -> ("StandardTemplate"=w382:string)  [unwired: 12 in, 1 out]
              }
            }
            n162 = case shown="False" w327 {
              tunnel: w337 -> [w347 w374]
              tunnel: w333 -> [w345 _]
              tunnel: [w344 w374] -> w310
              tunnel: w330 -> [w343 _]
              frame False {
                n163 = for {
                  N: 2 -> [_]
                  tunnel: w347 -> [w357]
                  tunnel: T7[] [] -> [w356]
                  tunnel: w345 -> [w350]
                  tunnel: [w354] -> w344
                  tunnel: w343 -> [w355]
                  i -> [w352]
                  stop <- w348 continue-if-true
                  n164 = Equal To 0?(x=w352) -> (x = 0?=w351:bool)
                  n165 = And(x=w350, y=w351) -> (x .and. y?=w349:bool)
                  n166 = for {
                    tunnel: w357 -> [w367] mode=indexing
                    shift-right: [w369] -> w354
                    shift-left: w356 -> [w368]
                    tunnel: w355 -> [w365]
                    tunnel: w349 -> [w361]
                    n167 = Unbundle By Name(w367) -> ("OnlySubClassTemplate"=w362:bool, "CanDeriveFromTheseTemplateIDs"=w366:string[])
                    n168 = Search 1D Array(1D array=w366, element=w365) -> (index of element=w359:i32)  [unwired: 1 in]
                    n169 = Compound Arithmetic op=AND(invert w361, invert w362) -> (w363:bool)
                    n170 = Greater Or Equal To 0?(x=w359) -> (x >= 0?=w360:bool)
                    n171 = Compound Arithmetic op=AND(w361, w360) -> (w358:bool)
                    n172 = Or(x=w363, y=w358) -> (x .or. y?=w364:bool)
                    n173 = case shown="True" w364 {
                      tunnel: w368 -> [w370 w373]
                      tunnel: [w370 w371] -> w369
                      tunnel: w367 -> [_ w372]
                      frame False {
                      }
                      frame True {
                        n174 = Build Array (concatenate)(w373, w372) -> (w371:T7[])
                      }
                    }
                  }
                  n175 = Array Size(array=w354) -> (size(s)=w353:i32)
                  n176 = Equal To 0?(x=w353) -> (x = 0?=w348:bool)
                }
              }
              frame True {
              }
            }
            n177 = Index Array(array=w310) -> (element=w309:T7)  [unwired: 1 in]
            n178 = Unbundle By Name(w309) -> ("TemplateIdName"=w308:string)
            n179 = call <resource>:"BaseProvider_ActorFramework_FindTemplates.vi"("MainClassemplateID"=w308, "FilterOnProviders"=w319, "DeriveFromClassRef"=w323) -> ("Array"=w322:T7[])  [unwired: 7 in, 1 out]
            n180 = Build Array (concatenate)(w322, w310) -> (w321:T7[])
            n181 = Array Size(array=w321) -> (size(s)=w332:i32)
            n182 = call <resource>:"DialogCreateClass_FilterAndOrderClassTemplates.vi"("error in (no error)"=w306, "AllTemplatesForThisProvider/InheritanceType(Base/Sub)"=w321) -> ("error out"=w305:errorcluster, "NewOrderIndex"=w304:i32[], "FilteredTemplates"=w307:T7[])  [unwired: 7 in]
            n183 = Bundle By Name(cluster=w320, "Templates"=w321, "ClassTemplateIndex"=w304) -> (w339:T10)
            n184 = for {
              tunnel: w307 -> [w379] mode=indexing
              tunnel: [w378] -> w335 mode=indexing
              tunnel: [w377] -> w331 mode=indexing
              tunnel: [w376] -> w325 mode=indexing
              tunnel: [w375] -> w318 mode=indexing
              n185 = Unbundle(w379) -> ("TemplateIdName"=w377:string, "TemplateUserDialogName"=w378:string, "ClassSuffix"=w376:string, "LvLibTemplate"=w375:bool)  [unwired: 3 out]
            }
            n186 = case shown="Default" w332 {
              tunnel: ["ChangeTheStartPath?" w390] -> w340
              tunnel: w326 -> [_ w388]
              frame Default {
              }
              frame 0 {
                n187 = case shown="False" w388 {
                  tunnel: ["ChangeTheStartPath?" "Exit"] -> w390
                  frame False {
                  }
                  frame True {
                  }
                }
                n188 = One Button Dialog(message="This class provider don't\nhave a sub class template\nto use when deriving for\nthe selected class.") -> ()  [unwired: 1 in, 1 out]
              }
            }
            n189 = Search 1D Array(1D array=w331, element=w330) -> (index of element=w329:i32)  [unwired: 1 in]
            n190 = property on="_ClassType" class="LstBox (strict)"("Value"=-1 ("_ClassType")) -> (error out=w311:errorcluster)  [unwired: 2 in, 1 out]
            n191 = Max & Min(x=w329, y=0 ("Class Type")) -> (max(x,y)=w317:i32)  [unwired: 1 out]
            n192 = Index Array(array=w325, index=w317) -> (element=w324:string)
            n193 = Index Array(array=w318, index=w317) -> (element=w316:bool)
            n194 = property on="_ClassType" class="LstBox (strict)"(error in=w311, "Item Names"=w335, "Val(Sgnl)"=w317) -> ()  [unwired: 1 in, 2 out]
            n195 = case shown="Default" w324 {
              selector: w324 -> [_ w341]
              frame "" {
              }
              frame Default {
                n196 = property on="_ClassFolderSuffix" class="Str"("Val(Sgnl)"=w341) -> ()  [unwired: 2 in, 2 out]
              }
            }
            n197 = Select(t="Library folder (The lvlib file will be saved in this directory)", s=w316, f=w313) -> (s? t:f=w314:string)
            n198 = property on="_ClassFolder" class="Path"("Caption.Text"=w314) -> ()  [unwired: 2 in, 2 out]
          }
          frame "ChangeTheStartPath?" {
            n199 = Unbundle By Name(w401) -> ("StartFolder"=w395:path, "DeriveFromClassRef"=w399:refnum<vi>)
            n200 = Not A Number/Path/Refnum?(number/path/refnum=w399) -> (NaN/Path/Refnum?=w396:bool)
            n201 = case shown="False" w396 {
              tunnel: w399 -> [w407 _]
              tunnel: [w408 _] -> w398
              tunnel: [w411 _] -> w394
              frame False {
                w405 = "Actor Framework.lvlib:Actor.lvclass" ("y")
                n202 = property class="LVClassLibrary"(reference=w407) -> ("Parent"=w418:refnum<vi>)  [unwired: 1 in, 2 out]
                n203 = call <resource>:"GDSLvClass_GetRootBaseClass.vi"("ViRef/Path,LvClassRef/Path"=w407, "Don'tOpenReference"=FALSE, "LimitToSpecificProviderTypeOfSameType(True)"=FALSE) -> ("RootBaseClassRef"=w419:refnum<vi>)  [unwired: 11 in, 5 out]
                n204 = property class="LVClassLibrary"(reference=w419) -> (reference out=w420:refnum<vi>, "QualifiedName"=w422:string)  [unwired: 1 in, 1 out]
                n205 = property class="LVClassLibrary"(reference=w407) -> ("QualifiedName"=w406:string)  [unwired: 1 in, 2 out]
                n206 = property class="ProjectItem"(reference=w418) -> (reference out=w414:refnum<vi>, error out=w415:errorcluster, "Type String"=w417:string, "Path"=w413:path)  [unwired: 1 in]
                n207 = Equal?(x=w407, y=w420) -> (x = y?=w421:bool)
                n208 = Equal?(x=w422, y=w405) -> (x = y?=w410:bool)
                n209 = Not Equal?(x=w405, y=w406) -> (x != y?=w404:bool)
                n210 = case shown="False" w421 {
                  tunnel: w420 -> [w425 _]
                  frame False {
                    n211 = Close Reference(reference=w425) -> ()  [unwired: 1 in, 1 out]
                  }
                  frame True {
                  }
                }
                n212 = Strip Path(path=w413) -> (stripped path=w412:path)  [unwired: 1 out]
                n213 = Equal?(x=w417, y="Library") -> (x = y?=w409:bool)
                n214 = Close Reference(reference=w414, error in (no error)=w415) -> ()  [unwired: 1 out]
                n215 = Strip Path(path=w412) -> (stripped path=w411:path)  [unwired: 1 out]
                n216 = Compound Arithmetic op=AND(w410, w404, w409) -> (w408:bool)
              }
              frame True {
              }
            }
            n217 = local read "_ClassName"() -> (w393:string)
            n218 = Select(t=w394, s=w398, f=w395) -> (s? t:f=w400:path)
            n219 = case shown="Default" w393 {
              selector: w393 -> [w403 _]
              frame Default {
                n220 = property on="_ClassName" class="Str"("Val(Sgnl)"=w403) -> ()  [unwired: 2 in, 2 out]
              }
              frame "" {
              }
            }
            n221 = property on="_ClassFolder" class="Path"("StartPath"=w400, "Value"=w400) -> ()  [unwired: 2 in, 2 out]
          }
          frame "GetClassInfo" {
          }
          frame "", "Idle" {
            n222 = local read "_ClassFolder"() -> (w444:path)
            n223 = Unbundle By Name(w434) -> ("Templates"=w429:T7[], "ClassTemplateIndex"=w432:i32[])
            n224 = local read "_ClassName"() -> (w447:string)
            n225 = local read "_ClassType"() -> (w446:i32)
            n226 = local read "_ClassType"() -> (w431:i32)
            n227 = List Folder(path=w444, pattern="*.lvclass") -> (filenames=w442:string[])  [unwired: 2 in, 3 out]
            n228 = Index Array(array=w432, index=w431) -> (element=w430:i32)
            n229 = Empty String/Path?(string/path=w444) -> (empty?=w449:bool)
            n230 = Array Size(array=w442) -> (size(s)=w441:i32)
            n231 = Empty String/Path?(string/path=w447) -> (empty?=w448:bool)
            n232 = Less Than 0?(x=w446) -> (x < 0?=w445:bool)
            n233 = Greater Than 0?(x=w441) -> (x > 0?=w440:bool)
            "DupPath" <- w440
            n234 = Index Array(array=w429, index=w430) -> (element=w435:T7)
            n235 = Compound Arithmetic op=OR(w440, w449, w448, w445) -> (w450:bool)
            n236 = Select(t=u8 2, s=w450, f=u8 0 ("Disabled")) -> (s? t:f=w453:u8)
            n237 = Unbundle By Name(w435) -> ("LvLibTemplate"=w433:bool)
            n238 = property on="_CreateClass" class="Bool"("Disabled"=w453) -> ()  [unwired: 2 in, 2 out]
            n239 = event shown="[16] \"InterfaceFilter\": Value Change" {
              selector: _ -> [_ _ _ _ _ _ _ _ _ _ _ _ _ _ _ _ _ _ _ _ _ _]
              dyn-events: _ -> [_ _ _ _ _ _ _ _ _ _ _ _ _ _ _ _ _ _ _ _ _ _]
              timeout: _ -> [_ _ _ _ _ _ _ _ _ _ _ _ _ _ _ _ _ _ _ _ _ _]
              tunnel: ["Exit" _ "Exit" "Idle" "Exit" "GetClassTemplateToUse" "Idle" w526 "Idle" "UpdateTemplates" _ "Idle" "Idle" "Idle" "Idle" w737 "UpdateInterfaceList" _ "Idle" "Idle" "Idle" "Idle"] -> w455
              tunnel: [TRUE _ w498 _ FALSE ("Cancel") _ _ _ _ _ _ _ _ _ _ _ _ _ _ _ _ _] -> w456
              tunnel: w434 -> [_ w470 _ _ _ _ _ w522 w572 _ _ w599 w611 w652 _ w742 _ _ _ _ _ _]
              tunnel: w439 -> [_ _ _ _ _ _ _ _ _ _ _ _ _ _ _ _ _ _ _ _ _ _]
              tunnel: w434 -> [w458 w472 w497 w500 w507 w509 w511 w525 w574 w588 w594 w600 w614 w654 w702 w739 w759 w765 w766 w774 w789 w799]
              tunnel: [w458 w467 w497 w500 w506 w509 w511 w524 w574 w588 w594 w600 w614 w654 w702 w738 w759 w765 w766 w774 w789 w799] -> w438
              tunnel: w437 -> [_ _ _ _ _ _ _ w521 _ _ _ _ _ _ _ _ _ _ _ _ _ _]
              tunnel: w436 -> [_ _ _ _ _ _ _ _ w566 _ _ _ _ _ _ _ _ _ _ _ _ _]
              tunnel: w433 -> [_ _ _ _ _ _ _ _ _ _ _ _ _ _ w701 _ _ _ _ _ w781 _]
              tunnel: w429 -> [_ _ _ _ _ _ _ _ _ w586 _ _ _ _ _ _ _ _ _ _ _ _]
              event "_Cancel": Value Change {
                n240 = event-data() -> ()  [unwired: 1 in, 2 out]
              }
              event Panel Resize {
                n241 = event-data() -> ("OldBnds"=w468:T6, "NewBnds"=w462:T6)  [unwired: 1 in]
                n242 = Unbundle By Name(w470) -> ("StartBnds"=w461:T6, "OldBnds"=w469:T6, "BondsChanged"=w465:bool)
                n243 = property class="VI"() -> ("FP.State"=w463:T21)  [unwired: 2 in, 2 out]
                n244 = Equal?(x=w468, y=w462) -> (x = y?=w471:bool)
                n245 = case shown="\"Maximized\"" w463 {
                  tunnel: w471 -> [_ w485]
                  tunnel: w469 -> [_ w484]
                  tunnel: w468 -> [w474 w483]
                  tunnel: [FALSE w482] -> w466
                  tunnel: w465 -> [_ w481]
                  tunnel: [w474 w480] -> w464
                  tunnel: w462 -> [w476 _]
                  tunnel: w461 -> [w475 _]
                  frame "Maximized" {
                    n246 = Unbundle By Name(w476) -> ("Top"=w477:i16, "Bottom"=w478:i16)
                    n247 = Bundle By Name(cluster=w475, "Top"=w477, "Bottom"=w478) -> (w479:T6)
                    n248 = property class="VI"("Front Panel.PanelBounds"=w479) -> ()  [unwired: 2 in, 2 out]
                  }
                  frame "Standard", Default {
                    n249 = case shown="False" w485 {
                      tunnel: w483 -> [w487 w491]
                      tunnel: [w488 w491] -> w480
                      tunnel: w484 -> [w489 w492]
                      tunnel: [TRUE FALSE] -> w482
                      tunnel: w481 -> [w486 _]
                      frame False {
                        n250 = Select(t=w489, s=w486, f=w487) -> (s? t:f=w488:T6)
                      }
                      frame True {
                        n251 = Unbundle By Name(w491) -> ("Top"=w496:i16, "Bottom"=w495:i16)
                        n252 = Bundle By Name(cluster=w492, "Top"=w496, "Bottom"=w495) -> (w494:T6)
                        n253 = property class="VI"("Front Panel.PanelBounds"=w494) -> ()  [unwired: 2 in, 2 out]
                      }
                    }
                  }
                }
                n254 = Bundle By Name(cluster=w472, "OldBnds"=w464, "BondsChanged"=w466) -> (w467:T10)
              }
              event Panel Close? {
                w498 = TRUE
                n255 = event-data() -> ()  [unwired: 1 in, 2 out]
                n256 = event-data("Discard?"=w498) -> ()  [unwired: 1 in, 1 out]
              }
              event "Help": Value Change {
                n257 = event-data() -> ()  [unwired: 1 in, 2 out]
                n258 = call <resource>:"GOOP_HelpMain.vi"() -> ()  [unwired: 12 in]
              }
              event "_CurrentClassProvider": Value Change {
                n259 = event-data() -> ()  [unwired: 1 in, 2 out]
                n260 = property on="_CurrentClassProvider" class="Ring (strict)"() -> ("Strings []"=w505:string[])  [unwired: 2 in, 2 out]
                n261 = Index Array(array=w505, index="_CurrentClassProvider") -> (element=w503:string)
                n262 = Bundle By Name(cluster=w507, "ChangeProviderTo"=w503) -> (w506:T10)
              }
              event "_CreateClass": Value Change {
                n263 = event-data() -> ()  [unwired: 1 in, 2 out]
              }
              event "_ClassDescription": Value Change {
                n264 = event-data() -> ()  [unwired: 1 in, 2 out]
              }
              event "AddDesignPattern": Value Change {
                w515 = i16 386  # Width of Design Pattern Pane
                n265 = event-data() -> ()  [unwired: 1 in, 2 out]
                n266 = Unbundle By Name(w522) -> ("DesignPatternsVisible"=w516:bool)
                n267 = disable-structure shown="Enabled" {
                  disable-tunnel: w516 -> [w535 _]
                  disable-tunnel: w522 -> [w534 _]
                  disable-tunnel: w521 -> [w527 _]
                  frame Disabled {
                    n268 = property class="VI"() -> ("Front Panel.PanelBounds"=w528:T6)  [unwired: 2 in, 2 out]
                    n269 = Unbundle By Name(w534) -> ("DPDescriptions"=w533:string[])
                    n270 = Unbundle By Name(w527) -> ("Right"=w538:i16, "Bottom"=w537:i16)
                    n271 = Array Size(array=w533) -> (size(s)=w532:i32)
                    n272 = Bundle("Right"=w538, "Bottom"=w537) -> (w536:cluster{"Right":i16, "Bottom":i16})  [unwired: 1 in]
                    n273 = case shown="True" w535 {
                      tunnel: [w546 w552] -> w540
                      tunnel: [w545 w550] -> w539
                      tunnel: w536 -> [w544 w551]
                      tunnel: w528 -> [w543 w549]
                      tunnel: w527 -> [w542 w548]
                      tunnel: [w541 w547] -> w529
                      frame False {
                        n274 = Add(x=w546, y=w544) -> (x+y=w545:cluster{"Right":i16, "Bottom":i16})
                        n275 = Add(x=w543, y=w542) -> (x+y=w541:T6)
                      }
                      frame True {
                        n276 = Subtract(x=w552, y=w551) -> (x-y=w550:cluster{"Right":i16, "Bottom":i16})
                        n277 = Subtract(x=w549, y=w548) -> (x-y=w547:T6)
                      }
                    }
                    n278 = Initialize Array(37, w532) -> (w530:i32[])
                    n279 = property on="DesignPatternList" class="LstBox (strict)"("Item Symbols"=w530) -> ()  [unwired: 2 in, 2 out]
                    n280 = property class="VI"("Front Panel.PanelBounds"=w529) -> ()  [unwired: 2 in, 2 out]
                  }
                  frame Enabled {
                  }
                }
                n281 = Not(x=w516) -> (.not. x?=w523:bool)
                n282 = Bundle By Name(cluster=w525, "DesignPatternsVisible"=w523) -> (w524:T10)
                n283 = property class="VI"() -> ("Front Panel.PanelBounds"=w519:T6)  [unwired: 2 in, 2 out]
                n284 = case shown="False" w523 {
                  tunnel: ["Idle" "GetDesignPatterns"] -> w526
                  frame False {
                  }
                  frame True {
                  }
                }
                n285 = Negate(x=w515) -> (-x=w514:i16)
                n286 = Unbundle By Name(w519) -> ("Right"=w520:i16)
                n287 = Select(t=w514, s=w516, f=w515) -> (s? t:f=w513:i16)
                n288 = Add(x=w520, y=w513) -> (x+y=w517:i16)
                n289 = Bundle By Name(cluster=w519, "Right"=w517) -> (w518:T6)
                n290 = property class="VI"("Front Panel.PanelBounds"=w518) -> ()  [unwired: 2 in, 2 out]
              }
              event "_ClassType": Value Change {
                n291 = event-data() -> ()  [unwired: 1 in, 2 out]
                n292 = Unbundle By Name(w572) -> ("Templates"=w571:T7[], "ClassFolderSuffix"=w568:string, "LLB_Allowed"=w559:bool, "ClassTemplateIndex"=w557:i32[])
                n293 = property on="_ClassFolderSuffix" class="Str"() -> (error out=w564:errorcluster, "Value"=w561:string)  [unwired: 2 in, 1 out]
                n294 = Index Array(array=w557, index="_ClassType") -> (element=w555:i32)
                n295 = Index Array(array=w571, index=w555) -> (element=w570:T7)
                n296 = Unbundle By Name(w570) -> ("ClassSuffix"=w569:string, "LvLibTemplate"=w560:bool)
                n297 = case shown="\"\"" w569 {
                  selector: w569 -> [_ w585]
                  tunnel: w568 -> [w584 _]
                  tunnel: [w584 w585] -> w563
                  frame "" {
                  }
                  frame Default {
                  }
                }
                n298 = Not Equal?(x=w561, y=w563) -> (x != y?=w562:bool)
                n299 = case shown="True" w562 {
                  tunnel: w561 -> [_ w579]
                  frame False {
                  }
                  frame True {
                    n300 = local read "_ClassFolder"() -> (w578:path)
                    n301 = Concatenate Strings(w579, "$" ("string")) -> (w582:string)
                    n302 = Strip Path(path=w578) -> (stripped path=w580:path, name=w583:string)
                    n303 = Match Pattern(string=w583, regular expression=w582) -> (before substring=w577:string)  [unwired: 1 in, 3 out]
                    n304 = Build Path(base path=w580, name or relative path=w577) -> (appended path=w576:path)
                    n305 = local write "_ClassFolder"(w576) -> ()
                  }
                }
                n306 = Select(t="Library folder (The lvlib file will be saved in this directory)", s=w560, f=w566) -> (s? t:f=w567:string)
                n307 = Compound Arithmetic op=AND(invert w560, w559) -> (w558:bool)
                n308 = property on="_ClassFolder" class="Path"("Caption.Text"=w567) -> ()  [unwired: 2 in, 2 out]
                n309 = property on="_UseLLB" class="Bool (strict)"("Visible"=w558) -> ()  [unwired: 2 in, 2 out]
                n310 = property on="_ClassFolderSuffix" class="Str"(error in=w564, "Val(Sgnl)"=w563) -> ()  [unwired: 1 in, 2 out]
                n311 = case shown="False" w558 {
                  frame False {
                    n312 = local write "_UseLLB"(FALSE ("_UseLLB")) -> ()
                  }
                  frame True {
                  }
                }
              }
              event "ModifyTemplates": Value Change {
                n313 = event-data() -> ()  [unwired: 1 in, 6 out]
                n314 = call <resource>:"DialogCreateClass_HandleTemplatesDialog.vi"("AllTemplatesForThisProvider/InheritanceType(Base/Sub)"=w586) -> ()  [unwired: 10 in, 1 out]
              }
              event Value Change {
                n315 = event-data() -> ()  [unwired: 1 in, 6 out]
                n316 = call <resource>:"BaseProvider_ConfigurationMemory.vi"() -> ("WireConfigurationOut"=w590:T22, "IconOut"=w589:string, "error out"=w593:errorcluster)  [unwired: 13 in, 4 out]
                n317 = call <resource>:"BaseProvider_ConfigurationMemory.vi"("WireConfiguration"=w590, "Icon"=w589, "error in (no error)"=w593, "Action"=enum16{"Read", "Load", "Save", "Set"}."Save", "PatternIn"="ConnectorPanePattern") -> ()  [unwired: 8 in, 7 out]
              }
              event "DesignPatternList": Value Change {
                n318 = event-data() -> ()  [unwired: 1 in, 2 out]
                n319 = Unbundle By Name(w599) -> ("DPDescriptions"=w598:string[])
                n320 = Index Array(array=w598, index="DesignPatternList") -> (element=→"DesignPatternDescription":string)
              }
              event "DesignPatternList": Double Click {
                n321 = event-data() -> ("Row"=w602:i32)  [unwired: 1 in]
                n322 = Unbundle By Name(w611) -> ("DpDependencies"=w610:cluster{"DependenciesID":string[]}[], "DPs"=w603:string[])
                n323 = property on="DesignPatternList" class="LstBox (strict)"() -> ("Item Symbols"=w609:i32[])  [unwired: 2 in, 2 out]
                n324 = Index Array(array=w609, index=w602) -> (element=w608:i32)
                n325 = Equal?(x=w608, y=37) -> (x = y?=w605:bool)
                n326 = Index Array(array=w603, index=w602) -> (element=w601:string)
                n327 = case shown="True" w605 {
                  tunnel: w610 -> [w618 w639]
                  tunnel: w603 -> [_ w638]
                  tunnel: w602 -> [w617 w637]
                  tunnel: [w615 w633] -> w606
                  tunnel: [37 38] -> w604
                  tunnel: w601 -> [w619 _]
                  frame False {
                    # "Uncheck this any and other selected DP that is dependent on this DP"
                    n328 = Build Array(w617) -> (w616:i32[])
                    n329 = for {
                      tunnel: w619 -> [w625]
                      tunnel: w618 -> [w627] mode=indexing
                      shift-right: [w622] -> w615
                      shift-left: w616 -> [w623]
                      i -> [w621]
                      n330 = Unbundle(w627) -> ("DependenciesID"=w626:string[])
                      n331 = Search 1D Array(1D array=w626, element=w625) -> (index of element=w624:i32)  [unwired: 1 in]
                      n332 = case shown="0, Default" w624 {
                        tunnel: w623 -> [w630 w631]
                        tunnel: [w629 w631] -> w622
                        tunnel: w621 -> [w628 _]
                        frame 0, Default {
                          n333 = Build Array (concatenate)(w628, w630) -> (w629:i32[])
                        }
                        frame -1 {
                        }
                      }
                    }
                  }
                  frame True {
                    # "Check this Dp and all it's dependency DPs"
                    n334 = Index Array(array=w639, index=w637) -> (element=w636:cluster{"DependenciesID":string[]})
                    n335 = Unbundle(w636) -> ("DependenciesID"=w635:string[])
                    n336 = for {
                      tunnel: w638 -> [w642]
                      tunnel: w635 -> [w641] mode=indexing
                      tunnel: [w640] -> w634 mode=indexing
                      n337 = Search 1D Array(1D array=w642, element=w641) -> (index of element=w640:i32)  [unwired: 1 in]
                    }
                    n338 = Build Array (concatenate)(w634, w637) -> (w633:i32[])
                  }
                }
                n339 = for {
                  shift-right: [w646] -> w613
                  shift-left: w609 -> [w645]
                  tunnel: w606 -> [w644] mode=indexing
                  tunnel: w604 -> [w643]
                  n340 = in-place {
                    in-place-border: w643 -> [w647]
                    n341 = in-place-array #2(w645, w644) -> ()  [unwired: 1 out]
                    n342 = in-place-array #2(w647) -> (w646:i32[])  [unwired: 1 out]
                  }
                }
                n343 = property on="DesignPatternList" class="LstBox (strict)"("Item Symbols"=w613) -> ()  [unwired: 2 in, 2 out]
              }
              event "DesignPatternList": Mouse Down {
                n344 = event-data() -> ("CtlRef"=w651:refnum<vi>, "Coords"=w650:T24)  [unwired: 1 in]
                n345 = invoke class="LstBox (strict)" method="Point To Row"(reference=w651, "Point"=w650) -> ("Row"=w649:i32, "InGlyph"=w648:bool)  [unwired: 5 in, 5 out]
                n346 = case shown="True" w648 {
                  tunnel: w652 -> [_ w665]
                  tunnel: w649 -> [_ w655]
                  frame False {
                  }
                  frame True {
                    n347 = Unbundle By Name(w665) -> ("DpDependencies"=w664:cluster{"DependenciesID":string[]}[], "DPs"=w657:string[])
                    n348 = property on="DesignPatternList" class="LstBox (strict)"() -> ("Item Symbols"=w663:i32[])  [unwired: 2 in, 2 out]
                    n349 = Index Array(array=w657, index=w655) -> (element=w656:string)
                    n350 = Index Array(array=w663, index=w655) -> (element=w662:i32)
                    n351 = Equal?(x=w662, y=37) -> (x = y?=w659:bool)
                    n352 = case shown="True" w659 {
                      tunnel: w664 -> [w670 w691]
                      tunnel: w657 -> [_ w690]
                      tunnel: w655 -> [w669 w689]
                      tunnel: [w667 w685] -> w660
                      tunnel: [37 38] -> w658
                      tunnel: w656 -> [w671 _]
                      frame False {
                        # "Uncheck this any and other selected DP that is dependent on this DP"
                        n353 = Build Array(w669) -> (w668:i32[])
                        n354 = for {
                          tunnel: w671 -> [w677]
                          tunnel: w670 -> [w679] mode=indexing
                          shift-right: [w674] -> w667
                          shift-left: w668 -> [w675]
                          i -> [w673]
                          n355 = Unbundle(w679) -> ("DependenciesID"=w678:string[])
                          n356 = Search 1D Array(1D array=w678, element=w677) -> (index of element=w676:i32)  [unwired: 1 in]
                          n357 = case shown="0, Default" w676 {
                            tunnel: w675 -> [w682 w683]
                            tunnel: [w681 w683] -> w674
                            tunnel: w673 -> [w680 _]
                            frame 0, Default {
                              n358 = Build Array (concatenate)(w680, w682) -> (w681:i32[])
                            }
                            frame -1 {
                            }
                          }
                        }
                      }
                      frame True {
                        # "Check this Dp and all \nit's dependency DPs"
                        n359 = Index Array(array=w691, index=w689) -> (element=w688:cluster{"DependenciesID":string[]})
                        n360 = Unbundle(w688) -> ("DependenciesID"=w687:string[])
                        n361 = for {
                          tunnel: w690 -> [w694]
                          tunnel: w687 -> [w693] mode=indexing
                          tunnel: [w692] -> w686 mode=indexing
                          n362 = Search 1D Array(1D array=w694, element=w693) -> (index of element=w692:i32)  [unwired: 1 in]
                        }
                        n363 = Build Array (concatenate)(w686, w689) -> (w685:i32[])
                      }
                    }
                    n364 = for {
                      shift-right: [w698] -> w666
                      shift-left: w663 -> [w697]
                      tunnel: w660 -> [w696] mode=indexing
                      tunnel: w658 -> [w695]
                      n365 = in-place {
                        in-place-border: w695 -> [w699]
                        n366 = in-place-array #3(w697, w696) -> ()  [unwired: 1 out]
                        n367 = in-place-array #3(w699) -> (w698:i32[])  [unwired: 1 out]
                      }
                    }
                    n368 = property on="DesignPatternList" class="LstBox (strict)"("Item Symbols"=w666) -> ()  [unwired: 2 in, 2 out]
                  }
                }
              }
              event "_ClassName": Value Change {
                n369 = event-data() -> ("OldVal"=w705:string)  [unwired: 1 in]
                n370 = case shown="False" w701 {
                  tunnel: [w719 _] -> w700
                  frame False {
                    n371 = local read "_ClassFolderSuffix"() -> (w719:string)
                  }
                  frame True {
                  }
                }
                n372 = local read "_ClassFolder"() -> (w712:path)
                n373 = Concatenate Strings(w705, ".llb" ("t")) -> (w703:string)
                n374 = call <resource>:"GOOP300_RemoveUnwantedChars.vi"("StringIn"="_ClassName") -> ("StringOut"=w715:string)  [unwired: 10 in]
                n375 = Strip Path(path=w712) -> (stripped path=w713:path, name=w706:string)
                n376 = Concatenate Strings(w705, w700) -> (w714:string)
                n377 = local write "_ClassName"(w715) -> ()
                n378 = Equal?(x=w706, y=w714) -> (x = y?=w708:bool)
                n379 = Equal?(x=w706, y=w703) -> (x = y?=w707:bool)
                n380 = Or(x=w708, y=w707) -> (x .or. y?=w709:bool)
                n381 = Select(t=w713, s=w709, f=w712) -> (s? t:f=w711:path)
                n382 = local read "_UseLLB"() -> (w710:bool)
                n383 = case shown="Default" w715 {
                  selector: w715 -> [_ w725]
                  tunnel: [w720 w728] -> w718
                  tunnel: w700 -> [_ w723]
                  tunnel: w711 -> [w720 w726]
                  tunnel: w710 -> [_ w724]
                  frame "" {
                  }
                  frame Default {
                    n384 = Select(t=".llb", s=w724, f=w723) -> (s? t:f=w722:string)
                    n385 = Concatenate Strings(w725, w722) -> (w727:string)
                    n386 = Build Path(base path=w726, name or relative path=w727) -> (appended path=w728:path)
                  }
                }
                n387 = local write "_ClassFolder"(w718) -> ()
              }
              event "_SelectParentClass": Value Change {
                n388 = event-data() -> ()  [unwired: 1 in, 1 out]
                n389 = Unbundle By Name(w742) -> ("ClassPaths"=w733:path[], "DeriveFromClassRef"=w741:refnum<vi>, "ClassTags"=w729:string[], "BaseObjectTag"=w736:string)
                n390 = Not Equal?(x=w736, y="_SelectParentClass") -> (x != y?=w735:bool)
                n391 = for {
                  tunnel: w733 -> [w756] mode=indexing
                  tunnel: [w754] -> _ mode=indexing
                  n392 = Strip Path(path=w756) -> (name=w755:string)  [unwired: 1 out]
                  n393 = Match Pattern(string=w755, regular expression="\\2Elvclass$") -> (before substring=w754:string)  [unwired: 1 in, 3 out]
                }
                n394 = Close Reference(reference=w741) -> (error out=w740:errorcluster)  [unwired: 1 in]
                n395 = stacked-sequence {
                  tunnel: w740 -> [_]
                  tunnel: w733 -> [w757]
                  tunnel: [w757] -> w732
                  frame #0 {
                  }
                }
                n396 = Search 1D Array(1D array=w729, element="_SelectParentClass") -> (index of element=w730:i32)  [unwired: 1 in]
                n397 = Index Array(array=w732, index=w730) -> (element=w734:path)
                n398 = case shown="-1" w730 {
                  tunnel: w739 -> [w748 w751]
                  tunnel: [w747 w750] -> w738
                  tunnel: ["GetTemplates" "GetTemplates"] -> w737
                  tunnel: w735 -> [w745 _]
                  tunnel: w734 -> [w744 _]
                  frame 0, Default {
                    n399 = call <resource>:"GDSLvClass_OpenClass.vi"("ClassToOpen"=w744) -> ("LVClass.Open"=w743:refnum<vi>)  [unwired: 17 in, 1 out]
                    n400 = Bundle By Name(cluster=w748, "Derived"=w745, "DeriveFromClass"=w744, "DeriveFromClassRef"=w743) -> (w747:T10)
                  }
                  frame -1 {
                    n401 = Bundle By Name(cluster=w751, "Derived"=FALSE) -> (w750:T10)
                  }
                }
              }
              event "InterfaceFilter": Value Change {
                n402 = event-data() -> ()  [unwired: 1 in, 6 out]
              }
              event "_SelectInterfaceClass": Value Change {
                n403 = event-data() -> ()  [unwired: 1 in, 6 out]
                n404 = Empty Array?(array="_SelectInterfaceClass") -> (empty?=w763:bool)
                n405 = Select(t=T16."Disabled and Grayed Out" ("Disabled"), s=w763, f=T16."Enabled" ("Disabled")) -> (s? t:f=w761:T16)
                n406 = property on="CreateInterfaceMethods" class="Enum (strict)"("DisabledEnum"=w761) -> ()  [unwired: 2 in, 2 out]
              }
              event "_UseLLB": Value Change {
                n407 = event-data() -> ()  [unwired: 1 in, 2 out]
                n408 = Select(t=u8 2 ("Disabled"), s="_UseLLB", f=u8 0 ("Disabled")) -> (s? t:f=w770:u8)
                n409 = property on="_ClassName" class="Str"() -> ("Value"=w767:string)  [unwired: 2 in, 2 out]
                n410 = property on="_ClassFolderSuffix" class="Str"("Disabled"=w770) -> ()  [unwired: 2 in, 2 out]
                n411 = property on="_ClassName" class="Str"("Val(Sgnl)"=w767) -> ()  [unwired: 2 in, 2 out]
              }
              event "_HelpCreateClass": Value Change {
                n412 = event-data() -> ("NewVal"=w773:bool)  [unwired: 1 in]
                n413 = Control Help Window(1:w773) -> ()  [unwired: 1 in]
              }
              event "_ClassFolderSuffix", "TriggerSuffixChange": Value Change {
                n414 = event-data() -> ("OldVal"=w777:string)  [unwired: 1 in, 2 out]
                n415 = local read "_ClassFolder"() -> (w791:path)
                n416 = call <resource>:"GOOP300_RemoveUnwantedChars.vi"("StringIn"="_ClassFolderSuffix") -> ("StringOut"=w778:string)  [unwired: 10 in]
                n417 = local write "_ClassFolderSuffix"(w778) -> ()
                n418 = Strip Path(path=w791) -> (stripped path=w786:path, name=w788:string)
                n419 = Select(t="", s=w781, f=w778) -> (s? t:f=w780:string)
                n420 = Build Array(w778, w777) -> (w776:string[])
                n421 = local read "_ClassName"() -> (w783:string)
                n422 = for {
                  tunnel: w776 -> [w793] mode=indexing
                  shift-right: [w794] -> w787
                  shift-left: w788 -> [w797]
                  n423 = Concatenate Strings(w793, "$" ("string")) -> (w796:string)
                  n424 = Match Pattern(string=w797, regular expression=w796) -> (before substring=w794:string)  [unwired: 1 in, 3 out]
                }
                n425 = Empty String/Path?(string/path=w783) -> (empty?=w782:bool)
                n426 = Concatenate Strings(w787, w780) -> (w785:string)
                n427 = Build Path(base path=w786, name or relative path=w785) -> (appended path=w784:path)
                n428 = case shown="False" w782 {
                  tunnel: w784 -> [w798 _]
                  frame False {
                    n429 = local write "_ClassFolder"(w798) -> ()
                  }
                  frame True {
                  }
                }
              }
              event "_ClassFolder": Value Change {
                n430 = event-data() -> ()  [unwired: 1 in, 2 out]
                n431 = Strip Path(path="_ClassFolder") -> ()  [unwired: 2 out]
                n432 = property on="_ClassName" class="Str"() -> ("Value"=w800:string)  [unwired: 2 in, 2 out]
                n433 = property on="_ClassName" class="Str"("Val(Sgnl)"=w800) -> ()  [unwired: 2 in, 2 out]
              }
            }
            n434 = Bundle By Name(cluster=w438, "Cancel"=w456) -> (w454:T10)
          }
          frame "UpdateTemplates" {
            n435 = Unbundle By Name(w809) -> ("Templates"=w806:T7[], "ClassTemplateIndex"=w808:i32[])
            n436 = local read "_ClassType"() -> (w807:i32)
            n437 = Index Array(array=w808, index=w807) -> (element=w805:i32)
            n438 = Index Array(array=w806, index=w805) -> (element=w804:T7)
            n439 = Unbundle By Name(w804) -> ("TemplateIdName"=w803:string)
            n440 = call <resource>:"DialogCreateClass_FilterAndOrderClassTemplates.vi"("AllTemplatesForThisProvider/InheritanceType(Base/Sub)"=w806) -> ("NewOrderIndex"=w823:i32[], "FilteredTemplates"=w810:T7[])  [unwired: 8 in, 1 out]
            n441 = for {
              tunnel: w810 -> [w832] mode=indexing
              tunnel: [w831] -> w822 mode=indexing
              tunnel: [w830] -> w821 mode=indexing
              tunnel: [w829] -> w819 mode=indexing
              tunnel: [w828] -> w817 mode=indexing
              n442 = Unbundle(w832) -> ("TemplateIdName"=w830:string, "TemplateUserDialogName"=w831:string, "ClassSuffix"=w829:string, "LvLibTemplate"=w828:bool)  [unwired: 3 out]
            }
            n443 = Bundle By Name(cluster=w809, "ClassTemplateIndex"=w823) -> (w824:T10)
            n444 = Search 1D Array(1D array=w821, element=w803) -> (index of element=w820:i32)  [unwired: 1 in]
            n445 = Max & Min(x=w820, y=0 ("Class Type")) -> (max(x,y)=w816:i32)  [unwired: 1 out]
            n446 = Index Array(array=w819, index=w816) -> (element=w818:string)
            n447 = Index Array(array=w817, index=w816) -> (element=w815:bool)
            n448 = property on="_ClassType" class="LstBox (strict)"("Item Names"=w822, "Val(Sgnl)"=w816) -> ()  [unwired: 2 in, 2 out]
            n449 = case shown="Default" w818 {
              selector: w818 -> [_ w827]
              frame "" {
              }
              frame Default {
                n450 = property on="_ClassFolderSuffix" class="Str"("Val(Sgnl)"=w827) -> ()  [unwired: 2 in, 2 out]
              }
            }
            n451 = Select(t="Library folder (The lvlib file will be saved in this directory)", s=w815, f=w811) -> (s? t:f=w814:string)
            n452 = property on="_ClassFolder" class="Path"("Caption.Text"=w814) -> ()  [unwired: 2 in, 2 out]
          }
          frame "GetDesignPatterns" {
            w834 = string[] []
            n453 = Unbundle By Name(w838) -> ("ClassProviderName"=w849:string, "ClassTemplateUsed"=w848:string)  [unwired: 1 out]
            n454 = call <resource>:"BaseProvider_DesignPattern_GetPatterns.vi"("FilterOnProviders(Ignored If Empty)"=w849, "FilterOnTemplate(Ignored If Empty)"=w848, "error in (no error)"=w847) -> ("DesignPatterns"=w845:T25[], "error out"=w846:errorcluster)  [unwired: 15 in]
            n455 = for {
              tunnel: w845 -> [w863] mode=indexing
              shift-right: [w860] -> w839
              shift-left: w834 -> [w859]
              shift-right: [w858] -> w841
              shift-left: w834 -> [w857]
              shift-right: [w856] -> w843
              shift-left: i32[] [] -> [w855]
              shift-right: [w853] -> w835
              shift-left: cluster{"DependenciesID":string[]}[] [] -> [w854]
              shift-right: [w852] -> w833
              shift-left: w834 -> [w851]
              n456 = Unbundle By Name(w863) -> ("Type"=w861:string, "Patterns"=w862:T26)
              n457 = for {
                tunnel: w862 -> [w888] mode=indexing
                tunnel: w861 -> [w887]
                shift-right: [w883] -> w860
                shift-left: w859 -> [w882]
                shift-right: [w879] -> w858
                shift-left: w857 -> [w880]
                shift-right: [w876] -> w856
                shift-left: w855 -> [w875]
                shift-right: [w866] -> w853
                shift-left: w854 -> [w865]
                shift-right: [w869] -> w852
                shift-left: w851 -> [w868]
                n458 = Unbundle By Name(w888) -> ("ID"=w870:string, "Name"=w886:string, "Desc"=w872:string, "Version"=w884:string, "DependenciesID"=w864:string[])  [unwired: 1 out]
                n459 = Array Size(array=w864) -> (size(s)=w873:i32)
                n460 = case shown="1.." w873 {
                  tunnel: ["" w891] -> w871
                  tunnel: w864 -> [_ w890]
                  frame 0, Default {
                  }
                  frame 1.. {
                    n461 = Array To Spreadsheet String(delimiter (Tab)=", ", array=w890, 3:"%s" ("format string")) -> (spreadsheet string=w892:string)
                    n462 = Format Into String(format string="\nDependencies: %s", w892) -> (resulting string=w891:string)  [unwired: 2 in, 1 out]
                  }
                }
                n463 = Format Into String(format string="%s : %s", w887, w886) -> (resulting string=w877:string)  [unwired: 2 in, 1 out]
                n464 = Bundle("DependenciesID"=w864) -> (w867:cluster{"DependenciesID":string[]})  [unwired: 1 in]
                n465 = Format Into String(format string="%s%s\n[%s, version: %s]", w872, w871, w870, w884) -> (resulting string=w881:string)  [unwired: 2 in, 1 out]
                n466 = Build Array (concatenate)(w865, w867) -> (w866:cluster{"DependenciesID":string[]}[])
                n467 = Build Array (concatenate)(w868, w870) -> (w869:string[])
                n468 = Build Array (concatenate)(w880, w877) -> (w879:string[])
                n469 = Build Array (concatenate)(w882, w881) -> (w883:string[])
                n470 = Build Array (concatenate)(w875, 37) -> (w876:i32[])
              }
            }
            n471 = property on="DesignPatternList" class="LstBox (strict)"("Item Names"=w841, "Item Symbols"=w843, "Value"=-1 ("Design Patterns"), "SelColor"=u32 14342874) -> ()  [unwired: 2 in, 2 out]
            n472 = Bundle By Name(cluster=w838, "DPs"=w833, "DPDescriptions"=w839, "DpDependencies"=w835) -> (w837:T10)
          }
          frame "GetClassTemplateToUse" {
            n473 = Unbundle By Name(w899) -> ("ClassPaths"=w903:path[], "ClassTags"=w904:string[], "BaseClasses"=w924:path[])  [unwired: 1 out]
            n474 = Unbundle By Name(w899) -> ("Templates"=w922:T7[], "DesignPatternsVisible"=w918:bool)
            n475 = local read "_SelectParentClass"() -> (w905:string)
            n476 = Unbundle By Name(w899) -> ("Templates"=w911:T7[], "ClassTemplateIndex"=w902:i32[])
            n477 = local read "_ClassType"() -> (w901:i32)
            n478 = for {
              tunnel: w922 -> [w973] mode=indexing
              tunnel: [w972] -> w921 mode=indexing
              n479 = Unbundle By Name(w973) -> ("TemplateIdName"=w972:string)  [unwired: 1 out]
            }
            n480 = disable-structure shown="Enabled" {
              disable-tunnel: w924 -> [w933 _]
              disable-tunnel: [w932 w940] -> w923
              disable-tunnel: w905 -> [w928 w943]
              disable-tunnel: w904 -> [_ w944]
              disable-tunnel: w903 -> [_ w942]
              frame Disabled {
                n481 = for {
                  tunnel: w933 -> [w939] mode=indexing
                  tunnel: [w936] -> w935 mode=indexing
                  n482 = Strip Path(path=w939) -> (name=w938:string)  [unwired: 1 out]
                  n483 = Match Pattern(string=w938, regular expression="\\2E[Ll][Vv][Cc][Ll][Aa][Ss][Ss]$") -> (before substring=w936:string)  [unwired: 1 in, 3 out]
                }
                n484 = To Lower Case(string=w935) -> (all lower case string=w934:string[])
                n485 = Match Pattern(string=w928, regular expression="\\2E[Ll][Vv][Cc][Ll][Aa][Ss][Ss]$") -> (before substring=w927:string)  [unwired: 1 in, 3 out]
                n486 = To Lower Case(string=w927) -> (all lower case string=w930:string)
                n487 = Search 1D Array(1D array=w934, element=w930) -> (index of element=w931:i32)  [unwired: 1 in]
                n488 = Index Array(array=w933, index=w931) -> (element=w932:path)
              }
              frame Enabled {
                n489 = Search 1D Array(1D array=w944, element=w943) -> (index of element=w941:i32)  [unwired: 1 in]
                n490 = Index Array(array=w942, index=w941) -> (element=w940:path)
              }
            }
            n491 = case shown="True" w918 {
              tunnel: w899 -> [_ w963]
              tunnel: [_ w957] -> w919
              frame False {
              }
              frame True {
                n492 = property on="DesignPatternList" class="LstBox (strict)"() -> ("Item Symbols"=w962:i32[])  [unwired: 2 in, 2 out]
                n493 = Unbundle By Name(w963) -> ("DPs"=w959:string[])
                n494 = Equal?(x=w962, y=38) -> (x = y?=w960:bool[])
                n495 = for {
                  shift-right: [w964] -> w957
                  shift-left: string[] [] -> [w966]
                  tunnel: w960 -> [w967] mode=indexing
                  tunnel: w959 -> [w965] mode=indexing
                  n496 = case shown="True" w967 {
                    tunnel: w966 -> [w968 w971]
                    tunnel: w965 -> [_ w970]
                    tunnel: [w968 w969] -> w964
                    frame False {
                    }
                    frame True {
                      n497 = Build Array (concatenate)(w971, w970) -> (w969:string[])
                    }
                  }
                }
              }
            }
            n498 = Index Array(array=w902, index=w901) -> (element=w900:i32)
            n499 = Index Array(array=w911, index=w900) -> (element=w910:T7)
            n500 = Unbundle By Name(w910) -> ("ClassSuffix"=w907:string)
            n501 = Unbundle By Name(w899) -> ("ClassTemplateIndex"=w898:i32[])
            n502 = property on="_ClassType" class="LstBox (strict)"() -> ("Value"=w897:i32)  [unwired: 2 in, 2 out]
            n503 = Empty String/Path?(string/path=w907) -> (empty?=w908:bool)
            n504 = Index Array(array=w898, index=w897) -> (element=w896:i32)
            n505 = local read "_ClassFolderSuffix"() -> (w912:string)
            n506 = Index Array(array=w921, index=w896) -> (element=w920:string)
            n507 = call <resource>:"BaseProvider_IniFileSettings.vi"("Action"=enum16{"Read", "Load", "Save"}."Read") -> ("IniFileSettings"=w913:T20)  [unwired: 17 in, 1 out]
            n508 = Unbundle By Name(w913) -> ("ClassFolderSuffix"=w914:string)
            n509 = Not Equal?(x=w914, y=w912) -> (x != y?=w909:bool)
            n510 = And(x=w909, y=w908) -> (x .and. y?=w906:bool)
            n511 = case shown="False" w906 {
              tunnel: w917 -> [w945 w949]
              tunnel: [w945 w948] -> w916
              tunnel: w913 -> [_ w947]
              tunnel: w912 -> [_ w946]
              frame False {
              }
              frame True {
                n512 = case shown="Default" w946 {
                  selector: w946 -> [_ w951]
                  tunnel: w949 -> [w950 w955]
                  tunnel: [w950 w954] -> w948
                  tunnel: w947 -> [_ w953]
                  frame "_Actor", "_Msg" {
                  }
                  frame Default {
                    n513 = Bundle By Name(cluster=w953, "ClassFolderSuffix"=w951) -> (w952:T20)
                    n514 = call <resource>:"BaseProvider_IniFileSettings.vi"("IniFileSettings"=w952, "error in (no error)"=w955, "Action"=enum16{"Read", "Load", "Save"}."Save") -> ("error out"=w954:errorcluster)  [unwired: 15 in, 1 out]
                  }
                }
              }
            }
            n515 = Bundle By Name(cluster=w899, "ClassType(Template)"=w920, "DPs"=w919, "BaseClassToUse"=w923) -> (w926:T10)
          }
          frame "GetInterfaceSettings" {
            n516 = local read "_SelectInterfaceClass"() -> (w985:i32[])
            n517 = property on="_SelectInterfaceClass" class="MCListbox (strict)"() -> ("ItemNames"=w988:string[][])  [unwired: 2 in, 2 out]
            n518 = Unbundle By Name(w984) -> ("InterfaceInfo"=w982:T8[])
            n519 = Index Array(array=w988, index (col)=0 ("disabled index (col)")) -> (element=w986:string[])  [unwired: 1 in]
            n520 = for {
              tunnel: w982 -> [w994] mode=indexing
              tunnel: [w993] -> w983 mode=indexing
              n521 = Unbundle By Name(w994) -> ("Name(Short if no Conflicts)"=w993:string)
            }
            n522 = for {
              tunnel: w986 -> [w1002]
              tunnel: w985 -> [w1001] mode=indexing
              tunnel: w983 -> [w1000]
              tunnel: w982 -> [w998]
              tunnel: [w996] -> w975 mode=indexing
              tunnel: [w995] -> w974 mode=indexing
              n523 = Index Array(array=w1002, index=w1001) -> (element=w999:string)
              n524 = Search 1D Array(1D array=w1000, element=w999) -> (index of element=w997:i32)  [unwired: 1 in]
              n525 = Index Array(array=w998, index=w997) -> (element=w995:T8)
              n526 = Unbundle By Name(w995) -> ("Path"=w996:path)
            }
            n527 = local read "CreateInterfaceMethods"() -> (w977:T2)
            n528 = case shown="\"Create some interface methods\"" w977 {
              tunnel: [_ w992] -> w976
              tunnel: w974 -> [_ w991]
              frame Default {
              }
              frame "Create some interface methods" {
                n529 = call <resource>:"SelectMethodsOfInterfaces.vi"("InterfacePath"=w991) -> ("MethodsPerInterface(Empty=>All)"=w992:cluster{"Methods":string[]}[])  [unwired: 9 in, 1 out]
              }
            }
            n530 = Greater Or Equal?(x=w977, y=T2."Create some interface methods") -> (x >= y?=w978:bool)
            n531 = Bundle By Name(cluster=T3 {"InterfacePath"=[], "CreateMethods"=FALSE, "MethodsPerInterface(Empty=>All)"=[]} ("InterfaceToImplement"), "InterfacePath"=w975, "CreateMethods"=w978, "MethodsPerInterface(Empty=>All)"=w976) -> (→"InterfaceToImplement":T3)
          }
          frame "Error", Default {
          }
          frame "Exit" {
          }
        }
      }
      n532 = call <vilib>:"Clear Errors.vi"("error in (no error)"=w34) -> ("error out"=w33:errorcluster)  [unwired: 5 in, 1 out]
      n533 = call <resource>:"GDSString_AddStatesToQueue.vi"() -> ()  [unwired: 15 in, 1 out]
      n534 = property on="_ClassFolder" class="Path"(error in=w33, "Caption.Text"=w37) -> ()  [unwired: 1 in, 2 out]
    }
    frame Error {
    }
  }
  "Reference out" <- w29
  "error out" <- w31
  n535 = Generate User Event(user event=w8, event data cluster="Stop" ("Stop")) -> (user event out=w10:refnum<user-event>)  [unwired: 2 in, 1 out]
  n536 = Destroy User Event(user event=w10) -> ()  [unwired: 1 in, 1 out]
  n537 = stacked-sequence {
    tunnel: w27 -> [w1016]
    tunnel: [w1029] -> w26
    tunnel: [w1028] -> w25
    tunnel: [w1024] -> w22
    tunnel: [w1027] -> w24
    tunnel: [w1026] -> w23
    tunnel: [w1025] -> w21
    tunnel: [w1023] -> _
    tunnel: "ProjectItem Refnum" -> [w1020]
    tunnel: w17 -> [w1019]
    tunnel: [w1017] -> w16
    tunnel: [w1015] -> w15
    tunnel: [w1014] -> w14
    frame #0 {
      n538 = Unbundle By Name(w1016) -> ("DesignPatternsVisible"=w1018:bool, "Cancel"=w1029:bool, "BaseClassToUse"=w1024:path, "ClassType(Template)"=w1025:string, "DeriveFromClassRef"=w1022:refnum<vi>)
      n539 = case shown="True" w1018 {
        tunnel: w1019 -> [_ w1030]
        frame False {
        }
        frame True {
          n540 = property class="VI"() -> ("Front Panel.PanelBounds"=w1032:T6)  [unwired: 2 in, 2 out]
          n541 = Subtract(x=w1032, y=w1030) -> (x-y=w1031:T6)
          n542 = property class="VI"("Front Panel.PanelBounds"=w1031) -> ()  [unwired: 2 in, 2 out]
        }
      }
      n543 = local read "_ClassFolder"() -> (w1028:path)
      n544 = local read "_ClassName"() -> (w1027:string)
      n545 = local read "_ClassDescription"() -> (w1026:string)
      n546 = local read "_ClassFolderSuffix"() -> (w1014:string)
      n547 = Unbundle By Name(w1016) -> ("ChangeProviderTo"=w1015:string)
      n548 = Not Equal?(x=w1022, y=w1020) -> (x != y?=w1021:bool)
      n549 = Unbundle By Name(w1016) -> ("DPs"=w1017:string[])
      n550 = case shown="True" w1021 {
        tunnel: [_ w1034] -> w1023
        tunnel: w1022 -> [_ w1033]
        frame False {
        }
        frame True {
          n551 = Close Reference(reference=w1033) -> (error out=w1034:errorcluster)  [unwired: 1 in]
        }
      }
    }
  }
  "Cancelled" <- w26
  "DesignPatternsToAddAfterCreation" <- w16
  "ChangeProviderRequested" <- w15
  n552 = Bundle By Name(cluster=T4 {"ClassName"="", "ClassFolder"=path "", "ClassDescription"="", "ClassTemplateOptions"="", "BaseClass(ProjectStringPath or LvClassFilePath)"=variant, "ExtraCreateParameters"=variant, "FolderSuffix"=""} ("CreateClassData"), "ClassFolder"=w25, "ClassName"=w24, "ClassDescription"=w23, "BaseClass(ProjectStringPath or LvClassFilePath)"=w22, "ClassTemplateOptions"=w21, "FolderSuffix"=w14) -> (→"CreateClassData":T4)
